vi "AS3_Spektrometer.vi"() -> ()   [LabVIEW 2013]
uses:
  subVIs_AS3_Spektrometer/ADC.vi
  subVIs_AS3_Spektrometer/readoutport.vi
panel:
  in  "Integration Time [s] 2":dbl=0.1
  in  "x-axis spectrum":cluster{dbl, dbl}(slide)={0.0, 3.6363636363636362} scale=0.0..10.0
  out "Camera NOT yet ready":bool
  in  "Leave Program":bool
  in  "Tab Control":T1(tab)=enum."Spectrum"
  in  "Autoscale Temperature":bool
  out "Temperature":cluster{dbl[], dbl[]}(graph)={[0.0, 0.25, 0.5, 0.75, 1.0, 1.25, 1.5, 1.75], [-30.0, -30.0, -30.0, -30.0, -30.0, -30.0, -30.0, -30.0]}
  in  "Temperature [°C]":dbl=-30.0
  out "Current Temperature [°C]":dbl=-30.0
  in  "Read Temperature":bool
  in  "stop 1":bool
  in  "Maximum Temperature Scale":dbl=-20.0
  in  "Minimum Temperature Scale":dbl=-40.0
  in  "Plot last 10 Seconds only":bool
  out "pixel scale":dbl[](array[numeric])=[0.0, 1.0, 2.0, 3.0, 4.0, 5.0, 6.0, 7.0, 8.0, 9.0, 10.0, 11.0, 12.0, 13.0, 14.0, 15.0, 16.0, 17.0, 18.0, 19.0, 20.0, 21.0, 22.0, 23.0, 24.0, 25.0, 26.0, 27.0, 28.0, 29.0, 30.0, 31.0, 32.0, 33.0, 34.0, 35.0, 36.0, 37.0, 38.0, 39.0, 40.0, 41.0, 42.0, 43.0, 44.0, 45.0, 46.0, 47.0, 48.0, 49.0, 50.0, 51.0, 52.0, 53.0, 54.0, 55.0, 56.0, 57.0, 58.0, 59.0, 60.0, 61.0, 62.0, 63.0, 64.0, 65.0, 66.0, 67.0, 68.0, 69.0, 70.0, 71.0, 72.0, 73.0, 74.0, 75.0, 76.0, 77.0, 78.0, 79.0, 80.0, 81.0, 82.0, 83.0, 84.0, 85.0, 86.0, 87.0, 88.0, 89.0, 90.0, 91.0, 92.0, 93.0, 94.0, 95.0, 96.0, 97.0, 98.0, 99.0, 100.0, 101.0, 102.0, 103.0, 104.0, 105.0, 106.0, 107.0, 108.0, 109.0, 110.0, 111.0, 112.0, 113.0, 114.0, 115.0, 116.0, 117.0, 118.0, 119.0, 120.0, 121.0, 122.0, 123.0, 124.0, 125.0, 126.0, 127.0, 128.0, 129.0, 130.0, 131.0, 132.0, 133.0, 134.0, 135.0, 136.0, 137.0, 138.0, 139.0, 140.0, 141.0, 142.0, 143.0, 144.0, 145.0, 146.0, 147.0, 148.0, 149.0, 150.0, 151.0, 152.0, 153.0, 154.0, 155.0, 156.0, 157.0, 158.0, 159.0, 160.0, 161.0, 162.0, 163.0, 164.0, 165.0, 166.0, 167.0, 168.0, 169.0, 170.0, 171.0, 172.0, 173.0, 174.0, 175.0, 176.0, 177.0, 178.0, 179.0, 180.0, 181.0, 182.0, 183.0, 184.0, 185.0, 186.0, 187.0, 188.0, 189.0, 190.0, 191.0, 192.0, 193.0, 194.0, 195.0, 196.0, 197.0, 198.0, 199.0, 200.0, 201.0, 202.0, 203.0, 204.0, 205.0, 206.0, 207.0, 208.0, 209.0, 210.0, 211.0, 212.0, 213.0, 214.0, 215.0, 216.0, 217.0, 218.0, 219.0, 220.0, 221.0, 222.0, 223.0, 224.0, 225.0, 226.0, 227.0, 228.0, 229.0, 230.0, 231.0, 232.0, 233.0, 234.0, 235.0, 236.0, 237.0, 238.0, 239.0, 240.0, 241.0, 242.0, 243.0, 244.0, 245.0, 246.0, 247.0, 248.0, 249.0, 250.0, 251.0, 252.0, 253.0, 254.0, 255.0, 256.0, 257.0, 258.0, 259.0, 260.0, 261.0, 262.0, 263.0, 264.0, 265.0, 266.0, 267.0, 268.0, 269.0, 270.0, 271.0, 272.0, 273.0, 274.0, 275.0, 276.0, 277.0, 278.0, 279.0, 280.0, 281.0, 282.0, 283.0, 284.0, 285.0, 286.0, 287.0, 288.0, 289.0, 290.0, 291.0, 292.0, 293.0, 294.0, 295.0, 296.0, 297.0, 298.0, 299.0, 300.0, 301.0, 302.0, 303.0, 304.0, 305.0, 306.0, 307.0, 308.0, 309.0, 310.0, 311.0, 312.0, 313.0, 314.0, 315.0, 316.0, 317.0, 318.0, 319.0, 320.0, 321.0, 322.0, 323.0, 324.0, 325.0, 326.0, 327.0, 328.0, 329.0, 330.0, 331.0, 332.0, 333.0, 334.0, 335.0, 336.0, 337.0, 338.0, 339.0, 340.0, 341.0, 342.0, 343.0, 344.0, 345.0, 346.0, 347.0, 348.0, 349.0, 350.0, 351.0, 352.0, 353.0, 354.0, 355.0, 356.0, 357.0, 358.0, 359.0, 360.0, 361.0, 362.0, 363.0, 364.0, 365.0, 366.0, 367.0, 368.0, 369.0, 370.0, 371.0, 372.0, 373.0, 374.0, 375.0, 376.0, 377.0, 378.0, 379.0, 380.0, 381.0, 382.0, 383.0, 384.0, 385.0, 386.0, 387.0, 388.0, 389.0, 390.0, 391.0, 392.0, 393.0, 394.0, 395.0, 396.0, 397.0, 398.0, 399.0, 400.0, 401.0, 402.0, 403.0, 404.0, 405.0, 406.0, 407.0, 408.0, 409.0, 410.0, 411.0, 412.0, 413.0, 414.0, 415.0, 416.0, 417.0, 418.0, 419.0, 420.0, 421.0, 422.0, 423.0, 424.0, 425.0, 426.0, 427.0, 428.0, 429.0, 430.0, 431.0, 432.0, 433.0, 434.0, 435.0, 436.0, 437.0, 438.0, 439.0, 440.0, 441.0, 442.0, 443.0, 444.0, 445.0, 446.0, 447.0, 448.0, 449.0, 450.0, 451.0, 452.0, 453.0, 454.0, 455.0, 456.0, 457.0, 458.0, 459.0, 460.0, 461.0, 462.0, 463.0, 464.0, 465.0, 466.0, 467.0, 468.0, 469.0, 470.0, 471.0, 472.0, 473.0, 474.0, 475.0, 476.0, 477.0, 478.0, 479.0, 480.0, 481.0, 482.0, 483.0, 484.0, 485.0, 486.0, 487.0, 488.0, 489.0, 490.0, 491.0, 492.0, 493.0, 494.0, 495.0, 496.0, 497.0, 498.0, 499.0, 500.0, 501.0, 502.0, 503.0, 504.0, 505.0, 506.0, 507.0, 508.0, 509.0, 510.0, 511.0, 512.0, 513.0, 514.0, 515.0, 516.0, 517.0, 518.0, 519.0, 520.0, 521.0, 522.0, 523.0, 524.0, 525.0, 526.0, 527.0, 528.0, 529.0, 530.0, 531.0, 532.0, 533.0, 534.0, 535.0, 536.0, 537.0, 538.0, 539.0, 540.0, 541.0, 542.0, 543.0, 544.0, 545.0, 546.0, 547.0, 548.0, 549.0, 550.0, 551.0, 552.0, 553.0, 554.0, 555.0, 556.0, 557.0, 558.0, 559.0, 560.0, 561.0, 562.0, 563.0, 564.0, 565.0, 566.0, 567.0, 568.0, 569.0, 570.0, 571.0, 572.0, 573.0, 574.0, 575.0, 576.0, 577.0, 578.0, 579.0, 580.0, 581.0, 582.0, 583.0, 584.0, 585.0, 586.0, 587.0, 588.0, 589.0, 590.0, 591.0, 592.0, 593.0, 594.0, 595.0, 596.0, 597.0, 598.0, 599.0, 600.0, 601.0, 602.0, 603.0, 604.0, 605.0, 606.0, 607.0, 608.0, 609.0, 610.0, 611.0, 612.0, 613.0, 614.0, 615.0, 616.0, 617.0, 618.0, 619.0, 620.0, 621.0, 622.0, 623.0, 624.0, 625.0, 626.0, 627.0, 628.0, 629.0, 630.0, 631.0, 632.0, 633.0, 634.0, 635.0, 636.0, 637.0, 638.0, 639.0, 640.0, 641.0, 642.0, 643.0, 644.0, 645.0, 646.0, 647.0, 648.0, 649.0, 650.0, 651.0, 652.0, 653.0, 654.0, 655.0, 656.0, 657.0, 658.0, 659.0, 660.0, 661.0, 662.0, 663.0, 664.0, 665.0, 666.0, 667.0, 668.0, 669.0, 670.0, 671.0, 672.0, 673.0, 674.0, 675.0, 676.0, 677.0, 678.0, 679.0, 680.0, 681.0, 682.0, 683.0, 684.0, 685.0, 686.0, 687.0, 688.0, 689.0, 690.0, 691.0, 692.0, 693.0, 694.0, 695.0, 696.0, 697.0, 698.0, 699.0, 700.0, 701.0, 702.0, 703.0, 704.0, 705.0, 706.0, 707.0, 708.0, 709.0, 710.0, 711.0, 712.0, 713.0, 714.0, 715.0, 716.0, 717.0, 718.0, 719.0, 720.0, 721.0, 722.0, 723.0, 724.0, 725.0, 726.0, 727.0, 728.0, 729.0, 730.0, 731.0, 732.0, 733.0, 734.0, 735.0, 736.0, 737.0, 738.0, 739.0, 740.0, 741.0, 742.0, 743.0, 744.0, 745.0, 746.0, 747.0, 748.0, 749.0, 750.0, 751.0, 752.0, 753.0, 754.0, 755.0, 756.0, 757.0, 758.0, 759.0, 760.0, 761.0, 762.0, 763.0, 764.0, 765.0, 766.0, 767.0, 768.0, 769.0, 770.0, 771.0, 772.0, 773.0, 774.0, 775.0, 776.0, 777.0, 778.0, 779.0, 780.0, 781.0, 782.0, 783.0, 784.0, 785.0, 786.0, 787.0, 788.0, 789.0, 790.0, 791.0, 792.0, 793.0, 794.0, 795.0, 796.0, 797.0, 798.0, 799.0, 800.0, 801.0, 802.0, 803.0, 804.0, 805.0, 806.0, 807.0, 808.0, 809.0, 810.0, 811.0, 812.0, 813.0, 814.0, 815.0, 816.0, 817.0, 818.0, 819.0, 820.0, 821.0, 822.0, 823.0, 824.0, 825.0, 826.0, 827.0, 828.0, 829.0, 830.0, 831.0, 832.0, 833.0, 834.0, 835.0, 836.0, 837.0, 838.0, 839.0, 840.0, 841.0, 842.0, 843.0, 844.0, 845.0, 846.0, 847.0, 848.0, 849.0, 850.0, 851.0, 852.0, 853.0, 854.0, 855.0, 856.0, 857.0, 858.0, 859.0, 860.0, 861.0, 862.0, 863.0, 864.0, 865.0, 866.0, 867.0, 868.0, 869.0, 870.0, 871.0, 872.0, 873.0, 874.0, 875.0, 876.0, 877.0, 878.0, 879.0, 880.0, 881.0, 882.0, 883.0, 884.0, 885.0, 886.0, 887.0, 888.0, 889.0, 890.0, 891.0, 892.0, 893.0, 894.0, 895.0, 896.0, 897.0, 898.0, 899.0, 900.0, 901.0, 902.0, 903.0, 904.0, 905.0, 906.0, 907.0, 908.0, 909.0, 910.0, 911.0, 912.0, 913.0, 914.0, 915.0, 916.0, 917.0, 918.0, 919.0, 920.0, 921.0, 922.0, 923.0, 924.0, 925.0, 926.0, 927.0, 928.0, 929.0, 930.0, 931.0, 932.0, 933.0, 934.0, 935.0, 936.0, 937.0, 938.0, 939.0, 940.0, 941.0, 942.0, 943.0, 944.0, 945.0, 946.0, 947.0, 948.0, 949.0, 950.0, 951.0, 952.0, 953.0, 954.0, 955.0, 956.0, 957.0, 958.0, 959.0, 960.0, 961.0, 962.0, 963.0, 964.0, 965.0, 966.0, 967.0, 968.0, 969.0, 970.0, 971.0, 972.0, 973.0, 974.0, 975.0, 976.0, 977.0, 978.0, 979.0, 980.0, 981.0, 982.0, 983.0, 984.0, 985.0, 986.0, 987.0, 988.0, 989.0, 990.0, 991.0, 992.0, 993.0, 994.0, 995.0, 996.0, 997.0, 998.0, 999.0, 1000.0, 1001.0, 1002.0, 1003.0, 1004.0, 1005.0, 1006.0, 1007.0, 1008.0, 1009.0, 1010.0, 1011.0, 1012.0, 1013.0, 1014.0, 1015.0, 1016.0, 1017.0, 1018.0, 1019.0, 1020.0, 1021.0, 1022.0, 1023.0, 1024.0, 1025.0, 1026.0, 1027.0, 1028.0, 1029.0, 1030.0, 1031.0, 1032.0, 1033.0, 1034.0, 1035.0, 1036.0, 1037.0, 1038.0, 1039.0, 1040.0, 1041.0, 1042.0, 1043.0, 1044.0, 1045.0, 1046.0, 1047.0, 1048.0, 1049.0, 1050.0, 1051.0, 1052.0, 1053.0, 1054.0, 1055.0, 1056.0, 1057.0, 1058.0, 1059.0, 1060.0, 1061.0, 1062.0, 1063.0, 1064.0, 1065.0, 1066.0, 1067.0, 1068.0, 1069.0, 1070.0, 1071.0, 1072.0, 1073.0, 1074.0, 1075.0, 1076.0, 1077.0, 1078.0, 1079.0, 1080.0, 1081.0, 1082.0, 1083.0, 1084.0, 1085.0, 1086.0, 1087.0, 1088.0, 1089.0, 1090.0, 1091.0, 1092.0, 1093.0, 1094.0, 1095.0, 1096.0, 1097.0, 1098.0, 1099.0, 1100.0, 1101.0, 1102.0, 1103.0, 1104.0, 1105.0, 1106.0, 1107.0, 1108.0, 1109.0, 1110.0, 1111.0, 1112.0, 1113.0, 1114.0, 1115.0, 1116.0, 1117.0, 1118.0, 1119.0, 1120.0, 1121.0, 1122.0, 1123.0, 1124.0, 1125.0, 1126.0, 1127.0, 1128.0, 1129.0, 1130.0, 1131.0, 1132.0, 1133.0, 1134.0, 1135.0, 1136.0, 1137.0, 1138.0, 1139.0, 1140.0, 1141.0, 1142.0, 1143.0, 1144.0, 1145.0, 1146.0, 1147.0, 1148.0, 1149.0, 1150.0, 1151.0, 1152.0, 1153.0, 1154.0, 1155.0, 1156.0, 1157.0, 1158.0, 1159.0, 1160.0, 1161.0, 1162.0, 1163.0, 1164.0, 1165.0, 1166.0, 1167.0, 1168.0, 1169.0, 1170.0, 1171.0, 1172.0, 1173.0, 1174.0, 1175.0, 1176.0, 1177.0, 1178.0, 1179.0, 1180.0, 1181.0, 1182.0, 1183.0, 1184.0, 1185.0, 1186.0, 1187.0, 1188.0, 1189.0, 1190.0, 1191.0, 1192.0, 1193.0, 1194.0, 1195.0, 1196.0, 1197.0, 1198.0, 1199.0, 1200.0, 1201.0, 1202.0, 1203.0, 1204.0, 1205.0, 1206.0, 1207.0, 1208.0, 1209.0, 1210.0, 1211.0, 1212.0, 1213.0, 1214.0, 1215.0, 1216.0, 1217.0, 1218.0, 1219.0, 1220.0, 1221.0, 1222.0, 1223.0, 1224.0, 1225.0, 1226.0, 1227.0, 1228.0, 1229.0, 1230.0, 1231.0, 1232.0, 1233.0, 1234.0, 1235.0, 1236.0, 1237.0, 1238.0, 1239.0, 1240.0, 1241.0, 1242.0, 1243.0, 1244.0, 1245.0, 1246.0, 1247.0, 1248.0, 1249.0, 1250.0, 1251.0, 1252.0, 1253.0, 1254.0, 1255.0, 1256.0, 1257.0, 1258.0, 1259.0, 1260.0, 1261.0, 1262.0, 1263.0, 1264.0, 1265.0, 1266.0, 1267.0, 1268.0, 1269.0, 1270.0, 1271.0, 1272.0, 1273.0, 1274.0, 1275.0, 1276.0, 1277.0, 1278.0, 1279.0, 1280.0, 1281.0, 1282.0, 1283.0, 1284.0, 1285.0, 1286.0, 1287.0, 1288.0, 1289.0, 1290.0, 1291.0, 1292.0, 1293.0, 1294.0, 1295.0, 1296.0, 1297.0, 1298.0, 1299.0, 1300.0, 1301.0, 1302.0, 1303.0, 1304.0, 1305.0, 1306.0, 1307.0, 1308.0, 1309.0, 1310.0, 1311.0, 1312.0, 1313.0, 1314.0, 1315.0, 1316.0, 1317.0, 1318.0, 1319.0, 1320.0, 1321.0, 1322.0, 1323.0, 1324.0, 1325.0, 1326.0, 1327.0, 1328.0, 1329.0, 1330.0, 1331.0, 1332.0, 1333.0, 1334.0, 1335.0, 1336.0, 1337.0, 1338.0, 1339.0]
  in  "Substract\nBackground":bool
  in  "Save Background":bool
  in  "Save Raw Data":bool
  in  "Change\nSettings":bool
  in  "Binning 1":u32(ring)=4 items=["1"=1, "2"=2, "4"=4, "10"=10]
  in  "Use Cursors":bool
  out "Current Loop":i32=1
  in  "Number of Averages":i32=1
  in  "Integration Time [s]":dbl=0.1
  in  "Scales of Full Chip Plot":T2={"X Max"=335.0, "Y Min"=1.0, "X Min"=1.0, "Y Max"=100.0}
  out "Full Chip Plot":dbl[][](graph)
  in  "stop 2":bool
  in  "Read Chip":bool
  out "ROI Parameters":T3={"X Start"=1, "X End"=1340, "Binning X"=4, "Y Start"=1, "Y End"=400, "Binning Y"=4}
  out "Plot Area":T4={"X min"=1.0, "Y min"=1.0, "X max"=335.0, "Y max"=100.0}
  out "Background Array":dbl[][](array[numeric])
  out "Binned Array 2":dbl[][](array[numeric])
  out "Binned Array 4":dbl[][](array[numeric])
  out "Binned Array 10":dbl[][](array[numeric])
  out "background\nspectrum":dbl[](array[numeric])=[4222.0, 3418.0, 3505.0, 3499.0, 3504.0, 3534.0, 3534.0, 3535.0, 3553.0, 3573.0, 3572.0, 3586.0, 3578.0, 3565.0, 3611.0, 3604.0, 3594.0, 3602.0, 3612.0, 3618.0, 3582.0, 3611.0, 3621.0, 3593.0, 3627.0, 3600.0, 3612.0, 3606.0, 3619.0, 3608.0, 3605.0, 3624.0, 3652.0, 3628.0, 3629.0, 3636.0, 3634.0, 3613.0, 3642.0, 3619.0, 3614.0, 3630.0, 3655.0, 3627.0, 3624.0, 3651.0, 3615.0, 3623.0, 3644.0, 3616.0, 3640.0, 3644.0, 3617.0, 3634.0, 3634.0, 3612.0, 3643.0, 3617.0, 3610.0, 3629.0, 3638.0, 3637.0, 3618.0, 3617.0, 3617.0, 3638.0, 3608.0, 3634.0, 3616.0, 3616.0, 3606.0, 3650.0, 3625.0, 3605.0, 3637.0, 3602.0, 3622.0, 3631.0, 3613.0, 3618.0, 3635.0, 3615.0, 3616.0, 3626.0, 3628.0, 3620.0, 3617.0, 3625.0, 3641.0, 3628.0, 3633.0, 3630.0, 3644.0, 3634.0, 3629.0, 3633.0, 3617.0, 3642.0, 3631.0, 3643.0, 3649.0, 3637.0, 3640.0, 3637.0, 3599.0, 3622.0, 3643.0, 3643.0, 3644.0, 3641.0, 3618.0, 3632.0, 3625.0, 3628.0, 3629.0, 3620.0, 3625.0, 3638.0, 3639.0, 3619.0, 3631.0, 3636.0, 3632.0, 3633.0, 3621.0, 3629.0, 3635.0, 3605.0, 3623.0, 3630.0, 3614.0, 3648.0, 3627.0, 3609.0, 3637.0, 3595.0, 3645.0, 3635.0, 3639.0, 3624.0, 3619.0, 3614.0, 3622.0, 3616.0, 3607.0, 3606.0, 3645.0, 3624.0, 3624.0, 3641.0, 3604.0, 3624.0, 3627.0, 3628.0, 3639.0, 3620.0, 3614.0, 3639.0, 3644.0, 3627.0, 3653.0, 3611.0, 3639.0, 3639.0, 3629.0, 3616.0, 3650.0, 3620.0, 3646.0, 3619.0, 3611.0, 3642.0, 3627.0, 3631.0, 3620.0, 3630.0, 3618.0, 3641.0, 3621.0, 3628.0, 3638.0, 3611.0, 3622.0, 3634.0, 3633.0, 3600.0, 3643.0, 3641.0, 3645.0, 3644.0, 3612.0, 3632.0, 3651.0, 3644.0, 3638.0, 3625.0, 3640.0, 3622.0, 3629.0, 3631.0, 3629.0, 3615.0, 3612.0, 3613.0, 3611.0, 3596.0, 3615.0, 3603.0, 3638.0, 3641.0, 3630.0, 3607.0, 3629.0, 3612.0, 3622.0, 3646.0, 3641.0, 3605.0, 3625.0, 3621.0, 3633.0, 3630.0, 3615.0, 3634.0, 3644.0, 3626.0, 3613.0, 3636.0, 3631.0, 3617.0, 3640.0, 3613.0, 3652.0, 3630.0, 3606.0, 3623.0, 3641.0, 3611.0, 3627.0, 3627.0, 3635.0, 3639.0, 3636.0, 3626.0, 3625.0, 3642.0, 3660.0, 3617.0, 3637.0, 3630.0, 3628.0, 3613.0, 3624.0, 3633.0, 3635.0, 3630.0, 3652.0, 3649.0, 3631.0, 3599.0, 3622.0, 3634.0, 3632.0, 3606.0, 3630.0, 3627.0, 3635.0, 3630.0, 3607.0, 3625.0, 3625.0, 3631.0, 3610.0, 3632.0, 3634.0, 3629.0, 3600.0, 3611.0, 3630.0, 3636.0, 3635.0, 3649.0, 3636.0, 3622.0, 3637.0, 3613.0, 3621.0, 3616.0, 3659.0, 3641.0, 3625.0, 3608.0, 3612.0, 3618.0, 3640.0, 3640.0, 3652.0, 3612.0, 3613.0, 3636.0, 3607.0, 3620.0, 3634.0, 3620.0, 3644.0, 3607.0, 3623.0, 3615.0, 3638.0, 3653.0, 3630.0, 3623.0, 3617.0, 3628.0, 3633.0, 3637.0, 3615.0, 3627.0, 3626.0, 3622.0, 3642.0, 3633.0, 3634.0, 3594.0, 3630.0, 3630.0, 3620.0, 3641.0, 3616.0, 3643.0, 3635.0, 3629.0, 3634.0, 3633.0, 3622.0, 3635.0, 3647.0, 3634.0, 3589.0, 3622.0, 3612.0, 3609.0, 3616.0, 3613.0, 3623.0, 3610.0, 3636.0, 3623.0, 3642.0, 3632.0, 3640.0, 3640.0, 3650.0, 3642.0, 3631.0, 3595.0, 3652.0, 3633.0, 3648.0, 3623.0, 3620.0, 3621.0, 3610.0, 3629.0, 3603.0, 3644.0, 3636.0, 3648.0, 3611.0, 3641.0, 3625.0, 3630.0, 3624.0, 3627.0, 3646.0, 3626.0, 3625.0, 3623.0, 3641.0, 3628.0, 3622.0, 3608.0, 3640.0, 3593.0, 3614.0, 3634.0, 3625.0, 3617.0, 3618.0, 3599.0, 3653.0, 3632.0, 3608.0, 3622.0, 3620.0, 3638.0, 3625.0, 3636.0, 3654.0, 3621.0, 3624.0, 3617.0, 3611.0, 3614.0, 3623.0, 3624.0, 3621.0, 3588.0, 3624.0, 3633.0, 3623.0, 3620.0, 3641.0, 3631.0, 3630.0, 3621.0, 3624.0, 3630.0, 3631.0, 3620.0, 3635.0, 3650.0, 3629.0, 3631.0, 3631.0, 3614.0, 3636.0, 3633.0, 3629.0, 3641.0, 3623.0, 3648.0, 3652.0, 3626.0, 3648.0, 3623.0, 3624.0, 3658.0, 3651.0, 3609.0, 3613.0, 3640.0, 3612.0, 3614.0, 3632.0, 3642.0, 3627.0, 3643.0, 3622.0, 3625.0, 3637.0, 3649.0, 3639.0, 3629.0, 3628.0, 3633.0, 3633.0, 3624.0, 3626.0, 3625.0, 3615.0, 3629.0, 3627.0, 3636.0, 3615.0, 3631.0, 3611.0, 3646.0, 3642.0, 3631.0, 3622.0, 3597.0, 3609.0, 3616.0, 3617.0, 3633.0, 3626.0, 3630.0, 3615.0, 3609.0, 3620.0, 3637.0, 3619.0, 3643.0, 3645.0, 3638.0, 3629.0, 3634.0, 3627.0, 3633.0, 3628.0, 3626.0, 3636.0, 3646.0, 3626.0, 3634.0, 3627.0, 3639.0, 3605.0, 3634.0, 3622.0, 3619.0, 3633.0, 3597.0, 3625.0, 3626.0, 3628.0, 3602.0, 3633.0, 3615.0, 3634.0, 3598.0, 3636.0, 3628.0, 3619.0, 3622.0, 3633.0, 3638.0, 3622.0, 3622.0, 3641.0, 3614.0, 3632.0, 3631.0, 3635.0, 3624.0, 3633.0, 3617.0, 3635.0, 3625.0, 3637.0, 3631.0, 3620.0, 3646.0, 3634.0, 3636.0, 3638.0, 3620.0, 3627.0, 3615.0, 3627.0, 3628.0, 3624.0, 3611.0, 3615.0, 3638.0, 3624.0, 3634.0, 3631.0, 3633.0, 3609.0, 3654.0, 3626.0, 3635.0, 3632.0, 3623.0, 3618.0, 3619.0, 3604.0, 3634.0, 3613.0, 3637.0, 3642.0, 3612.0, 3626.0, 3625.0, 3616.0, 3636.0, 3626.0, 3643.0, 3642.0, 3633.0, 3637.0, 3609.0, 3615.0, 3621.0, 3626.0, 3641.0, 3623.0, 3627.0, 3637.0, 3608.0, 3604.0, 3626.0, 3612.0, 3621.0, 3624.0, 3623.0, 3616.0, 3634.0, 3658.0, 3612.0, 3635.0, 3615.0, 3659.0, 3624.0, 3630.0, 3637.0, 3607.0, 3630.0, 3630.0, 3621.0, 3616.0, 3635.0, 3648.0, 3617.0, 3633.0, 3605.0, 3625.0, 3645.0, 3601.0, 3620.0, 3626.0, 3632.0, 3639.0, 3642.0, 3620.0, 3624.0, 3644.0, 3646.0, 3614.0, 3623.0, 3607.0, 3630.0, 3627.0, 3615.0, 3637.0, 3593.0, 3609.0, 3641.0, 3629.0, 3627.0, 3644.0, 3637.0, 3637.0, 3642.0, 3626.0, 3626.0, 3639.0, 3632.0, 3635.0, 3623.0, 3611.0, 3629.0, 3629.0, 3626.0, 3630.0, 3624.0, 3622.0, 3623.0, 3626.0, 3622.0, 3625.0, 3620.0, 3635.0, 3624.0, 3629.0, 3636.0, 3650.0, 3601.0, 3616.0, 3629.0, 3615.0, 3624.0, 3615.0, 3608.0, 3655.0, 3612.0, 3622.0, 3598.0, 3618.0, 3629.0, 3658.0, 3605.0, 3613.0, 3655.0, 3596.0, 3629.0, 3633.0, 3615.0, 3631.0, 3639.0, 3626.0, 3615.0, 3622.0, 3630.0, 3630.0, 3620.0, 3640.0, 3621.0, 3628.0, 3625.0, 3619.0, 3614.0, 3634.0, 3624.0, 3610.0, 3627.0, 3629.0, 3620.0, 3659.0, 3631.0, 3645.0, 3624.0, 3637.0, 3635.0, 3627.0, 3632.0, 3623.0, 3612.0, 3631.0, 3622.0, 3643.0, 3619.0, 3638.0, 3635.0, 3616.0, 3637.0, 3619.0, 3635.0, 3632.0, 3619.0, 3638.0, 3628.0, 3641.0, 3623.0, 3637.0, 3644.0, 3633.0, 3630.0, 3642.0, 3620.0, 3643.0, 3623.0, 3637.0, 3627.0, 3638.0, 3621.0, 3622.0, 3641.0, 3618.0, 3625.0, 3630.0, 3615.0, 3626.0, 3648.0, 3646.0, 3636.0, 3620.0, 3637.0, 3643.0, 3620.0, 3653.0, 3627.0, 3590.0, 3626.0, 3614.0, 3626.0, 3608.0, 3627.0, 3624.0, 3638.0, 3632.0, 3627.0, 3670.0, 3625.0, 3620.0, 3627.0, 3635.0, 3638.0, 3617.0, 3644.0, 3629.0, 3638.0, 3629.0, 3635.0, 3618.0, 3624.0, 3627.0, 3637.0, 3614.0, 3623.0, 3626.0, 3635.0, 3612.0, 3640.0, 3639.0, 3619.0, 3597.0, 3647.0, 3628.0, 3621.0, 3642.0, 3649.0, 3609.0, 3609.0, 3640.0, 3630.0, 3635.0, 3628.0, 3603.0, 3628.0, 3599.0, 3621.0, 3646.0, 3661.0, 3613.0, 3641.0, 3640.0, 3637.0, 3635.0, 3621.0, 3653.0, 3623.0, 3626.0, 3630.0, 3609.0, 3618.0, 3627.0, 3618.0, 3614.0, 3626.0, 3629.0, 3624.0, 3633.0, 3628.0, 3618.0, 3619.0, 3631.0, 3608.0, 3620.0, 3646.0, 3632.0, 3625.0, 3644.0, 3630.0, 3638.0, 3608.0, 3633.0, 3635.0, 3619.0, 3636.0, 3636.0, 3620.0, 3621.0, 3621.0, 3613.0, 3613.0, 3635.0, 3643.0, 3628.0, 3629.0, 3643.0, 3632.0, 3645.0, 3613.0, 3652.0, 3640.0, 3627.0, 3627.0, 3622.0, 3624.0, 3629.0, 3630.0, 3614.0, 3645.0, 3609.0, 3615.0, 3629.0, 3623.0, 3637.0, 3623.0, 3634.0, 3624.0, 3631.0, 3615.0, 3621.0, 3645.0, 3622.0, 3613.0, 3621.0, 3615.0, 3627.0, 3638.0, 3646.0, 3632.0, 3654.0, 3614.0, 3626.0, 3630.0, 3627.0, 3624.0, 3627.0, 3621.0, 3648.0, 3630.0, 3620.0, 3635.0, 3623.0, 3608.0, 3618.0, 3620.0, 3656.0, 3629.0, 3604.0, 3645.0, 3627.0, 3612.0, 3641.0, 3644.0, 3637.0, 3633.0, 3628.0, 3624.0, 3638.0, 3624.0, 3628.0, 3628.0, 3618.0, 3621.0, 3646.0, 3620.0, 3643.0, 3660.0, 3634.0, 3624.0, 3611.0, 3621.0, 3632.0, 3622.0, 3604.0, 3649.0, 3625.0, 3624.0, 3635.0, 3650.0, 3616.0, 3629.0, 3633.0, 3627.0, 3622.0, 3615.0, 3632.0, 3638.0, 3624.0, 3638.0, 3634.0, 3627.0, 3620.0, 3631.0, 3621.0, 3619.0, 3637.0, 3629.0, 3636.0, 3620.0, 3623.0, 3614.0, 3657.0, 3629.0, 3633.0, 3604.0, 3616.0, 3631.0, 3624.0, 3601.0, 3640.0, 3642.0, 3643.0, 3629.0, 3649.0, 3641.0, 3647.0, 3628.0, 3612.0, 3651.0, 3628.0, 3631.0, 3635.0, 3640.0, 3650.0, 3616.0, 3647.0, 3635.0, 3652.0, 3629.0, 3612.0, 3620.0, 3628.0, 3630.0, 3639.0, 3629.0, 3625.0, 3632.0, 3617.0, 3639.0, 3629.0, 3622.0, 3658.0, 3616.0, 3652.0, 3638.0, 3612.0, 3624.0, 3607.0, 3646.0, 3619.0, 3640.0, 3611.0, 3641.0, 3629.0, 3602.0, 3630.0, 3608.0, 3630.0, 3631.0, 3611.0, 3629.0, 3604.0, 3637.0, 3638.0, 3633.0, 3642.0, 3622.0, 3631.0, 3608.0, 3620.0, 3626.0, 3630.0, 3627.0, 3619.0, 3618.0, 3607.0, 3626.0, 3634.0, 3627.0, 3636.0, 3621.0, 3637.0, 3629.0, 3608.0, 3642.0, 3640.0, 3607.0, 3615.0, 3594.0, 3633.0, 3615.0, 3612.0, 3629.0, 3650.0, 3619.0, 3650.0, 3625.0, 3610.0, 3635.0, 3632.0, 3633.0, 3629.0, 3631.0, 3640.0, 3622.0, 3638.0, 3614.0, 3638.0, 3629.0, 3622.0, 3646.0, 3614.0, 3614.0, 3617.0, 3640.0, 3623.0, 3610.0, 3612.0, 3623.0, 3632.0, 3622.0, 3651.0, 3624.0, 3623.0, 3641.0, 3645.0, 3634.0, 3651.0, 3622.0, 3627.0, 3625.0, 3620.0, 3617.0, 3617.0, 3646.0, 3629.0, 3621.0, 3630.0, 3613.0, 3621.0, 3645.0, 3634.0, 3631.0, 3635.0, 3651.0, 3620.0, 3620.0, 3633.0, 3628.0, 3632.0, 3623.0, 3636.0, 3615.0, 3595.0, 3626.0, 3638.0, 3623.0, 3620.0, 3642.0, 3621.0, 3621.0, 3625.0, 3611.0, 3633.0, 3616.0, 3623.0, 3632.0, 3645.0, 3613.0, 3611.0, 3623.0, 3633.0, 3619.0, 3624.0, 3639.0, 3599.0, 3640.0, 3627.0, 3606.0, 3628.0, 3644.0, 3622.0, 3607.0, 3637.0, 3618.0, 3630.0, 3613.0, 3614.0, 3631.0, 3612.0, 3637.0, 3613.0, 3641.0, 3636.0, 3633.0, 3621.0, 3628.0, 3633.0, 3623.0, 3654.0, 3632.0, 3601.0, 3623.0, 3621.0, 3643.0, 3648.0, 3642.0, 3610.0, 3608.0, 3633.0, 3604.0, 3611.0, 3634.0, 3620.0, 3633.0, 3627.0, 3611.0, 3630.0, 3601.0, 3622.0, 3631.0, 3608.0, 3620.0, 3620.0, 3615.0, 3642.0, 3613.0, 3627.0, 3621.0, 3617.0, 3617.0, 3633.0, 3620.0, 3612.0, 3625.0, 3660.0, 3649.0, 3629.0, 3630.0, 3616.0, 3630.0, 3631.0, 3642.0, 3615.0, 3622.0, 3625.0, 3622.0, 3629.0, 3628.0, 3609.0, 3623.0, 3617.0, 3615.0, 3639.0, 3619.0, 3631.0, 3611.0, 3609.0, 3618.0, 3641.0, 3617.0, 3605.0, 3634.0, 3623.0, 3606.0, 3638.0, 3624.0, 3629.0, 3648.0, 3600.0, 3630.0, 3613.0, 3627.0, 3615.0, 3621.0, 3626.0, 3617.0, 3650.0, 3625.0, 3597.0, 3620.0, 3611.0, 3621.0, 3619.0, 3633.0, 3620.0, 3630.0, 3634.0, 3644.0, 3626.0, 3641.0, 3639.0, 3629.0, 3618.0, 3623.0, 3628.0, 3624.0, 3603.0, 3627.0, 3631.0, 3647.0, 3639.0, 3636.0, 3632.0, 3631.0, 3629.0, 3635.0, 3625.0, 3643.0, 3619.0, 3618.0, 3632.0, 3631.0, 3606.0, 3626.0, 3633.0, 3638.0, 3622.0, 3629.0, 3607.0, 3630.0, 3614.0, 3627.0, 3646.0, 3625.0, 3624.0, 3623.0, 3632.0, 3606.0, 3614.0, 3629.0, 3619.0, 3629.0, 3631.0, 3621.0, 3633.0, 3608.0, 3644.0, 3620.0, 3621.0, 3620.0, 3633.0, 3610.0, 3625.0, 3634.0, 3638.0, 3615.0, 3626.0, 3631.0, 3629.0, 3632.0, 3614.0, 3604.0, 3608.0, 3609.0, 3606.0, 3648.0, 3654.0, 3619.0, 3665.0, 3614.0, 3607.0, 3632.0, 3639.0, 3604.0, 3624.0, 3637.0, 3634.0, 3624.0, 3636.0, 3628.0, 3639.0, 3618.0, 3631.0, 3610.0, 3629.0, 3638.0, 3612.0, 3624.0, 3628.0, 3648.0, 3629.0]
  out "Index 2":u32=1
  out "Index 1":u32=1
  out "Image Handle":u32=1
  out "back":dbl[][](array[numeric])
  in  "Comment":string="MCP \nNe mbar"
  in  "Save to Logbook":bool
  in  "Autoscale":bool=TRUE
  in  "Use latest\nEnergy Scale":bool
  in  "New Calibration":bool
  out "already calibrated?":bool=TRUE
  in  "stop 3":bool
  in  "Start Calibration":bool
  in  "calibration spectra":u16(ring)=2 items=["current spectrum"=1, "averaged spectrum"=2, "background spectrum"=4]
  in  "Number of\nAverages":i32=3
  out "Current\nLoop":i32=2
  out "normalized spectra":cluster{dbl[], dbl[]}[](graph)
  in  "Calibrate":bool
  in  "First Edge [eV]":dbl=100.0
  in  "Second Edge [eV]":dbl=72.8
  in  "Save second spectrum for calibration":bool
  in  "Save first spectrum for calibration":bool
  out "current spectrum":cluster{"Value":dbl[], "Value":dbl[]}[](graph)
  out "background spectrum":cluster{"Value":dbl[], dbl[]}[](graph)
  out "averaged spectrum":T5(graph)
  in  "Substract\nBackground 2":bool
  out "Energy Scale in eV":dbl[](array[numeric])=[56.2886283295992, 56.36666666666666, 56.44470500373413, 56.52274334080158, 56.60078167786905, 56.67882001493652, 56.756858352003974, 56.83489668907144, 56.9129350261389, 56.990973363206365, 57.06901170027383, 57.147050037341295, 57.225088374408756, 57.303126711476224, 57.381165048543686, 57.45920338561115, 57.53724172267861, 57.61528005974607, 57.69331839681354, 57.771356733881, 57.84939507094846, 57.92743340801593, 58.00547174508339, 58.08351008215085, 58.16154841921832, 58.23958675628578, 58.31762509335324, 58.395663430420704, 58.473701767488166, 58.551740104555634, 58.629778441623095, 58.70781677869056, 58.785855115758025, 58.86389345282549, 58.94193178989295, 59.019970126960416, 59.09800846402788, 59.17604680109534, 59.25408513816281, 59.33212347523027, 59.41016181229773, 59.48820014936519, 59.56623848643265, 59.64427682350012, 59.72231516056758, 59.800353497635044, 59.87839183470251, 59.95643017176997, 60.034468508837435, 60.1125068459049, 60.190545182972365, 60.268583520039826, 60.34662185710729, 60.42466019417475, 60.50269853124222, 60.58073686830968, 60.65877520537714, 60.73681354244461, 60.81485187951207, 60.89289021657953, 60.970928553647, 61.04896689071446, 61.12700522778192, 61.20504356484938, 61.283081901916844, 61.36112023898431, 61.439158576051774, 61.517196913119236, 61.595235250186704, 61.673273587254165, 61.75131192432163, 61.829350261389095, 61.907388598456556, 61.98542693552402, 62.063465272591486, 62.14150360965895, 62.21954194672641, 62.29758028379387, 62.37561862086133, 62.4536569579288, 62.53169529499626, 62.60973363206372, 62.68777196913119, 62.76581030619865, 62.843848643266114, 62.92188698033358, 62.99992531740104, 63.077963654468505, 63.156001991535966, 63.23404032860343, 63.312078665670896, 63.39011700273836, 63.46815533980582, 63.54619367687329, 63.62423201394075, 63.70227035100821, 63.78030868807568, 63.85834702514314, 63.9363853622106, 64.01442369927807, 64.09246203634552, 64.17050037341299, 64.24853871048046, 64.32657704754791, 64.40461538461538, 64.48265372168285, 64.5606920587503, 64.63873039581776, 64.71676873288524, 64.7948070699527, 64.87284540702015, 64.95088374408762, 65.02892208115509, 65.10696041822254, 65.18499875529001, 65.26303709235748, 65.34107542942493, 65.4191137664924, 65.49715210355987, 65.57519044062732, 65.65322877769479, 65.73126711476226, 65.80930545182972, 65.88734378889718, 65.96538212596465, 66.0434204630321, 66.12145880009957, 66.19949713716704, 66.2775354742345, 66.35557381130195, 66.43361214836943, 66.51165048543689, 66.58968882250434, 66.66772715957183, 66.74576549663928, 66.82380383370673, 66.9018421707742, 66.97988050784167, 67.05791884490912, 67.1359571819766, 67.21399551904406, 67.29203385611152, 67.37007219317898, 67.44811053024645, 67.5261488673139, 67.60418720438138, 67.68222554144884, 67.7602638785163, 67.83830221558377, 67.91634055265123, 67.99437888971869, 68.07241722678616, 68.15045556385363, 68.22849390092108, 68.30653223798855, 68.384570575056, 68.46260891212347, 68.54064724919094, 68.6186855862584, 68.69672392332586, 68.77476226039332, 68.85280059746079, 68.93083893452825, 69.00887727159571, 69.08691560866318, 69.16495394573064, 69.2429922827981, 69.32103061986557, 69.39906895693304, 69.47710729400049, 69.55514563106796, 69.63318396813543, 69.71122230520288, 69.78926064227035, 69.86729897933782, 69.94533731640527, 70.02337565347274, 70.10141399054021, 70.17945232760766, 70.25749066467513, 70.33552900174259, 70.41356733881005, 70.49160567587751, 70.56964401294498, 70.64768235001245, 70.7257206870799, 70.80375902414737, 70.88179736121484, 70.95983569828229, 71.03787403534976, 71.11591237241723, 71.19395070948468, 71.27198904655215, 71.35002738361962, 71.42806572068707, 71.50610405775454, 71.58414239482201, 71.66218073188946, 71.74021906895693, 71.8182574060244, 71.89629574309186, 71.97433408015932, 72.05237241722678, 72.13041075429425, 72.20844909136171, 72.28648742842917, 72.36452576549664, 72.44256410256409, 72.52060243963156, 72.59864077669903, 72.67667911376648, 72.75471745083395, 72.83275578790142, 72.91079412496887, 72.98883246203634, 73.06687079910381, 73.14490913617126, 73.22294747323873, 73.3009858103062, 73.37902414737366, 73.45706248444112, 73.53510082150859, 73.61313915857605, 73.69117749564352, 73.76921583271098, 73.84725416977844, 73.9252925068459, 74.00333084391336, 74.08136918098083, 74.15940751804828, 74.23744585511575, 74.31548419218322, 74.39352252925067, 74.47156086631814, 74.54959920338561, 74.62763754045307, 74.70567587752053, 74.783714214588, 74.86175255165546, 74.93979088872292, 75.0178292257904, 75.09586756285785, 75.17390589992532, 75.25194423699278, 75.32998257406024, 75.40802091112771, 75.48605924819518, 75.56409758526263, 75.6421359223301, 75.72017425939757, 75.79821259646502, 75.87625093353249, 75.95428927059994, 76.03232760766741, 76.11036594473487, 76.18840428180233, 76.2664426188698, 76.34448095593726, 76.42251929300473, 76.5005576300722, 76.57859596713965, 76.65663430420712, 76.73467264127459, 76.81271097834204, 76.89074931540951, 76.96878765247698, 77.04682598954443, 77.1248643266119, 77.20290266367937, 77.28094100074682, 77.35897933781429, 77.43701767488176, 77.51505601194921, 77.59309434901668, 77.67113268608414, 77.7491710231516, 77.82720936021907, 77.90524769728653, 77.983286034354, 78.06132437142145, 78.13936270848892, 78.21740104555639, 78.29543938262384, 78.37347771969131, 78.45151605675878, 78.52955439382623, 78.6075927308937, 78.68563106796117, 78.76366940502862, 78.84170774209609, 78.91974607916356, 78.99778441623101, 79.07582275329848, 79.15386109036595, 79.2318994274334, 79.30993776450087, 79.38797610156834, 79.4660144386358, 79.54405277570326, 79.62209111277072, 79.70012944983819, 79.77816778690564, 79.85620612397311, 79.93424446104058, 80.01228279810803, 80.0903211351755, 80.16835947224297, 80.24639780931042, 80.32443614637789, 80.40247448344536, 80.48051282051281, 80.55855115758028, 80.63658949464775, 80.7146278317152, 80.79266616878267, 80.87070450585014, 80.9487428429176, 81.02678117998506, 81.10481951705253, 81.18285785411999, 81.26089619118746, 81.33893452825492, 81.41697286532238, 81.49501120238985, 81.5730495394573, 81.65108787652477, 81.72912621359222, 81.80716455065969, 81.88520288772716, 81.96324122479461, 82.04127956186208, 82.11931789892955, 82.197356235997, 82.27539457306447, 82.35343291013194, 82.4314712471994, 82.50950958426687, 82.58754792133433, 82.66558625840179, 82.74362459546926, 82.82166293253673, 82.89970126960418, 82.97773960667165, 83.05577794373912, 83.13381628080657, 83.21185461787404, 83.2898929549415, 83.36793129200896, 83.44596962907642, 83.52400796614388, 83.60204630321135, 83.6800846402788, 83.75812297734628, 83.83616131441374, 83.9141996514812, 83.99223798854867, 84.07027632561613, 84.14831466268359, 84.22635299975106, 84.30439133681853, 84.38242967388598, 84.46046801095345, 84.53850634802092, 84.61654468508837, 84.69458302215584, 84.77262135922331, 84.85065969629076, 84.92869803335823, 85.0067363704257, 85.08477470749315, 85.16281304456062, 85.24085138162808, 85.31888971869554, 85.39692805576301, 85.47496639283047, 85.55300472989794, 85.63104306696539, 85.70908140403286, 85.78711974110033, 85.86515807816778, 85.94319641523525, 86.02123475230272, 86.09927308937017, 86.17731142643764, 86.25534976350511, 86.33338810057256, 86.41142643764003, 86.4894647747075, 86.56750311177495, 86.64554144884242, 86.72357978590989, 86.80161812297735, 86.87965646004481, 86.95769479711228, 87.03573313417974, 87.1137714712472, 87.19180980831466, 87.26984814538213, 87.34788648244958, 87.42592481951705, 87.50396315658452, 87.58200149365197, 87.66003983071944, 87.73807816778691, 87.81611650485436, 87.89415484192183, 87.9721931789893, 88.05023151605675, 88.12826985312422, 88.20630819019169, 88.28434652725915, 88.36238486432661, 88.44042320139408, 88.51846153846154, 88.596499875529, 88.67453821259647, 88.75257654966393, 88.8306148867314, 88.90865322379886, 88.98669156086632, 89.06472989793379, 89.14276823500124, 89.22080657206871, 89.29884490913616, 89.37688324620363, 89.4549215832711, 89.53295992033856, 89.61099825740602, 89.68903659447349, 89.76707493154095, 89.84511326860842, 89.92315160567588, 90.00118994274334, 90.0792282798108, 90.15726661687827, 90.23530495394573, 90.3133432910132, 90.39138162808067, 90.46941996514812, 90.54745830221559, 90.62549663928306, 90.70353497635051, 90.78157331341798, 90.85961165048543, 90.9376499875529, 91.01568832462037, 91.09372666168782, 91.1717649987553, 91.24980333582275, 91.32784167289022, 91.40588000995768, 91.48391834702514, 91.5619566840926, 91.63999502116008, 91.71803335822753, 91.796071695295, 91.87411003236247, 91.95214836942992, 92.03018670649739, 92.10822504356486, 92.18626338063231, 92.26430171769978, 92.34234005476725, 92.4203783918347, 92.49841672890217, 92.57645506596964, 92.6544934030371, 92.73253174010456, 92.81057007717202, 92.88860841423949, 92.96664675130694, 93.04468508837441, 93.12272342544188, 93.20076176250933, 93.2788000995768, 93.35683843664427, 93.43487677371172, 93.51291511077919, 93.59095344784666, 93.66899178491411, 93.74703012198158, 93.82506845904905, 93.9031067961165, 93.98114513318397, 94.05918347025144, 94.1372218073189, 94.21526014438636, 94.29329848145383, 94.37133681852129, 94.44937515558875, 94.52741349265622, 94.60545182972368, 94.68349016679115, 94.7615285038586, 94.83956684092607, 94.91760517799352, 94.99564351506099, 95.07368185212846, 95.15172018919591, 95.22975852626338, 95.30779686333085, 95.3858352003983, 95.46387353746577, 95.54191187453324, 95.6199502116007, 95.69798854866816, 95.77602688573563, 95.85406522280309, 95.93210355987055, 96.01014189693802, 96.08818023400548, 96.16621857107295, 96.24425690814041, 96.32229524520787, 96.40033358227534, 96.47837191934279, 96.55641025641026, 96.63444859347773, 96.71248693054518, 96.79052526761265, 96.8685636046801, 96.94660194174757, 97.02464027881504, 97.1026786158825, 97.18071695294996, 97.25875529001743, 97.33679362708489, 97.41483196415236, 97.49287030121982, 97.57090863828728, 97.64894697535475, 97.72698531242222, 97.80502364948967, 97.88306198655714, 97.9611003236246, 98.03913866069206, 98.11717699775953, 98.195215334827, 98.27325367189445, 98.35129200896192, 98.42933034602937, 98.50736868309684, 98.5854070201643, 98.66344535723177, 98.74148369429923, 98.81952203136669, 98.89756036843416, 98.97559870550162, 99.05363704256908, 99.13167537963655, 99.20971371670402, 99.28775205377147, 99.36579039083894, 99.4438287279064, 99.52186706497386, 99.59990540204133, 99.6779437391088, 99.75598207617625, 99.83402041324372, 99.91205875031119, 99.99009708737864, 100.06813542444611, 100.14617376151358, 100.22421209858103, 100.3022504356485, 100.38028877271596, 100.45832710978343, 100.53636544685088, 100.61440378391835, 100.69244212098582, 100.77048045805327, 100.84851879512074, 100.92655713218821, 101.00459546925566, 101.08263380632313, 101.1606721433906, 101.23871048045805, 101.31674881752552, 101.39478715459299, 101.47282549166044, 101.55086382872791, 101.62890216579538, 101.70694050286284, 101.7849788399303, 101.86301717699777, 101.94105551406523, 102.0190938511327, 102.09713218820015, 102.17517052526762, 102.25320886233507, 102.33124719940254, 102.40928553647001, 102.48732387353746, 102.56536221060493, 102.6434005476724, 102.72143888473985, 102.79947722180732, 102.87751555887479, 102.95555389594224, 103.03359223300971, 103.11163057007718, 103.18966890714464, 103.2677072442121, 103.34574558127957, 103.42378391834703, 103.5018222554145, 103.57986059248196, 103.65789892954942, 103.73593726661689, 103.81397560368436, 103.89201394075181, 103.97005227781928, 104.04809061488673, 104.1261289519542, 104.20416728902165, 104.28220562608912, 104.36024396315659, 104.43828230022405, 104.51632063729151, 104.59435897435898, 104.67239731142644, 104.7504356484939, 104.82847398556137, 104.90651232262883, 104.9845506596963, 105.06258899676376, 105.14062733383122, 105.21866567089869, 105.29670400796616, 105.37474234503361, 105.45278068210108, 105.53081901916855, 105.608857356236, 105.68689569330346, 105.76493403037094, 105.84297236743839, 105.92101070450585, 105.99904904157333, 106.07708737864078, 106.15512571570824, 106.2331640527757, 106.31120238984317, 106.38924072691063, 106.4672790639781, 106.54531740104557, 106.62335573811302, 106.70139407518049, 106.77943241224796, 106.85747074931541, 106.93550908638288, 107.01354742345035, 107.0915857605178, 107.16962409758527, 107.24766243465274, 107.3257007717202, 107.40373910878766, 107.48177744585513, 107.55981578292258, 107.63785411999004, 107.71589245705752, 107.79393079412498, 107.87196913119243, 107.9500074682599, 108.02804580532737, 108.10608414239482, 108.18412247946229, 108.26216081652976, 108.34019915359721, 108.41823749066468, 108.49627582773215, 108.5743141647996, 108.65235250186707, 108.73039083893454, 108.808429176002, 108.88646751306946, 108.96450585013693, 109.04254418720438, 109.12058252427185, 109.19862086133932, 109.27665919840678, 109.35469753547423, 109.43273587254171, 109.51077420960917, 109.58881254667662, 109.6668508837441, 109.74488922081156, 109.82292755787901, 109.90096589494648, 109.97900423201395, 110.0570425690814, 110.13508090614887, 110.21311924321634, 110.2911575802838, 110.36919591735126, 110.44723425441873, 110.52527259148619, 110.60331092855365, 110.68134926562112, 110.75938760268858, 110.83742593975605, 110.91546427682351, 110.99350261389097, 111.07154095095844, 111.1495792880259, 111.22761762509336, 111.30565596216081, 111.3836942992283, 111.46173263629575, 111.5397709733632, 111.61780931043069, 111.69584764749814, 111.7738859845656, 111.85192432163306, 111.92996265870053, 112.00800099576799, 112.08603933283545, 112.16407766990292, 112.24211600697038, 112.32015434403785, 112.39819268110531, 112.47623101817277, 112.55426935524024, 112.6323076923077, 112.71034602937516, 112.78838436644263, 112.8664227035101, 112.94446104057755, 113.02249937764502, 113.10053771471249, 113.17857605177994, 113.2566143888474, 113.33465272591488, 113.41269106298233, 113.49072940004979, 113.56876773711726, 113.64680607418472, 113.72484441125218, 113.80288274831965, 113.88092108538711, 113.95895942245457, 114.03699775952204, 114.1150360965895, 114.19307443365696, 114.27111277072443, 114.3491511077919, 114.42718944485935, 114.50522778192682, 114.58326611899429, 114.66130445606174, 114.73934279312921, 114.81738113019668, 114.89541946726413, 114.97345780433159, 115.05149614139907, 115.12953447846652, 115.20757281553398, 115.28561115260146, 115.36364948966892, 115.44168782673637, 115.51972616380384, 115.5977645008713, 115.67580283793876, 115.75384117500623, 115.8318795120737, 115.90991784914115, 115.98795618620862, 116.06599452327609, 116.14403286034354, 116.22207119741101, 116.30010953447848, 116.37814787154593, 116.4561862086134, 116.53422454568087, 116.61226288274833, 116.6903012198158, 116.76833955688326, 116.84637789395072, 116.92441623101817, 117.00245456808565, 117.08049290515311, 117.15853124222056, 117.23656957928803, 117.3146079163555, 117.39264625342295, 117.47068459049042, 117.54872292755789, 117.62676126462534, 117.70479960169281, 117.78283793876028, 117.86087627582774, 117.9389146128952, 118.01695294996267, 118.09499128703013, 118.1730296240976, 118.25106796116506, 118.32910629823252, 118.40714463529999, 118.48518297236745, 118.56322130943491, 118.64125964650236, 118.71929798356985, 118.7973363206373, 118.87537465770475, 118.95341299477224, 119.03145133183969, 119.10948966890714, 119.18752800597461, 119.26556634304208, 119.34360468010954, 119.421643017177, 119.49968135424447, 119.57771969131193, 119.6557580283794, 119.73379636544686, 119.81183470251432, 119.88987303958179, 119.96791137664925, 120.04594971371671, 120.12398805078418, 120.20202638785165, 120.2800647249191, 120.35810306198657, 120.43614139905404, 120.51417973612149, 120.59221807318895, 120.67025641025643, 120.74829474732388, 120.82633308439134, 120.90437142145882, 120.98240975852627, 121.06044809559373, 121.1384864326612, 121.21652476972866, 121.29456310679612, 121.37260144386359, 121.45063978093106, 121.52867811799851, 121.60671645506598, 121.68475479213345, 121.7627931292009, 121.84083146626837, 121.91886980333584, 121.99690814040329, 122.07494647747076, 122.15298481453823, 122.23102315160568, 122.30906148867315, 122.38709982574062, 122.46513816280807, 122.54317649987553, 122.62121483694301, 122.69925317401047, 122.77729151107792, 122.85532984814539, 122.93336818521286, 123.01140652228031, 123.08944485934778, 123.16748319641525, 123.2455215334827, 123.32355987055017, 123.40159820761764, 123.47963654468509, 123.55767488175256, 123.63571321882003, 123.71375155588748, 123.79178989295495, 123.86982823002242, 123.94786656708987, 124.02590490415734, 124.10394324122481, 124.18198157829227, 124.26001991535972, 124.3380582524272, 124.41609658949466, 124.49413492656211, 124.5721732636296, 124.65021160069705, 124.7282499377645, 124.80628827483197, 124.88432661189944, 124.9623649489669, 125.04040328603436, 125.11844162310183, 125.19647996016928, 125.27451829723675, 125.35255663430422, 125.43059497137168, 125.50863330843914, 125.58667164550661, 125.66470998257407, 125.74274831964154, 125.820786656709, 125.89882499377646, 125.97686333084393, 126.0549016679114, 126.13294000497885, 126.2109783420463, 126.28901667911379, 126.36705501618124, 126.4450933532487, 126.52313169031616, 126.60117002738363, 126.67920836445109, 126.75724670151855, 126.83528503858602, 126.91332337565348, 126.99136171272094, 127.06940004978841, 127.14743838685587, 127.22547672392334, 127.3035150609908, 127.38155339805826, 127.45959173512573, 127.5376300721932, 127.61566840926065, 127.69370674632812, 127.77174508339559, 127.84978342046304, 127.9278217575305, 128.00586009459798, 128.08389843166543, 128.1619367687329, 128.23997510580037, 128.31801344286782, 128.39605177993528, 128.47409011700273, 128.5521284540702, 128.63016679113767, 128.70820512820512, 128.7862434652726, 128.86428180234006, 128.9423201394075, 129.020358476475, 129.09839681354245, 129.1764351506099, 129.2544734876774, 129.33251182474484, 129.4105501618123, 129.48858849887978, 129.56662683594723, 129.6446651730147, 129.72270351008217, 129.80074184714962, 129.87878018421708, 129.95681852128456, 130.03485685835201, 130.11289519541947, 130.19093353248695, 130.2689718695544, 130.34701020662186, 130.42504854368934, 130.5030868807568, 130.58112521782425, 130.65916355489173, 130.7372018919592, 130.81524022902664, 130.89327856609412, 130.97131690316158, 131.04935524022903, 131.12739357729652, 131.20543191436397, 131.28347025143142, 131.3615085884989, 131.43954692556636, 131.51758526263382, 131.5956235997013, 131.67366193676875, 131.7517002738362, 131.82973861090366, 131.90777694797114, 131.9858152850386, 132.06385362210605, 132.1418919591735, 132.219930296241, 132.29796863330844, 132.3760069703759, 132.45404530744338, 132.53208364451083, 132.6101219815783, 132.68816031864577, 132.76619865571323, 132.84423699278068, 132.92227532984816, 133.00031366691562, 133.07835200398307, 133.15639034105055, 133.234428678118, 133.31246701518546, 133.39050535225294, 133.4685436893204, 133.54658202638785, 133.62462036345534, 133.7026587005228, 133.78069703759024, 133.85873537465773, 133.93677371172518, 134.01481204879263, 134.09285038586012, 134.17088872292757, 134.24892705999503, 134.3269653970625, 134.40500373412996, 134.48304207119742, 134.5610804082649, 134.63911874533235, 134.7171570823998, 134.7951954194673, 134.87323375653474, 134.9512720936022, 135.02931043066968, 135.10734876773714, 135.1853871048046, 135.26342544187207, 135.34146377893953, 135.41950211600698, 135.49754045307444, 135.5755787901419, 135.65361712720937, 135.73165546427683, 135.80969380134428, 135.88773213841176, 135.96577047547922, 136.04380881254667, 136.12184714961415, 136.1998854866816, 136.27792382374906, 136.35596216081655, 136.434000497884, 136.51203883495145, 136.59007717201894, 136.6681155090864, 136.74615384615385, 136.82419218322133, 136.90223052028878, 136.98026885735624, 137.05830719442372, 137.13634553149117, 137.21438386855863, 137.2924222056261, 137.37046054269356, 137.44849887976102, 137.5265372168285, 137.60457555389596, 137.6826138909634, 137.7606522280309, 137.83869056509835, 137.9167289021658, 137.99476723923328, 138.07280557630074, 138.1508439133682, 138.22888225043567, 138.30692058750313, 138.38495892457058, 138.46299726163807, 138.54103559870552, 138.61907393577297, 138.69711227284046, 138.7751506099079, 138.85318894697537, 138.93122728404285, 139.00926562111027, 139.08730395817776, 139.16534229524524, 139.24338063231266, 139.32141896938015, 139.39945730644763, 139.47749564351506, 139.55553398058254, 139.63357231765002, 139.71161065471745, 139.78964899178493, 139.86768732885238, 139.94572566591984, 140.02376400298732, 140.10180234005477, 140.17984067712223, 140.2578790141897, 140.33591735125717, 140.41395568832462, 140.4919940253921, 140.57003236245956, 140.648070699527, 140.7261090365945, 140.80414737366195, 140.8821857107294, 140.96022404779688, 141.03826238486434, 141.1163007219318, 141.19433905899928, 141.27237739606673, 141.35041573313418, 141.42845407020167, 141.50649240726912, 141.58453074433658, 141.66256908140406, 141.7406074184715, 141.81864575553897, 141.89668409260645, 141.9747224296739, 142.05276076674136, 142.13079910380884, 142.2088374408763, 142.28687577794375, 142.36491411501123, 142.44295245207869, 142.52099078914614, 142.59902912621362, 142.67706746328105, 142.75510580034853, 142.833144137416, 142.91118247448344, 142.98922081155092, 143.0672591486184, 143.14529748568583, 143.2233358227533, 143.3013741598208, 143.37941249688822, 143.4574508339557, 143.53548917102316, 143.6135275080906, 143.6915658451581, 143.76960418222555, 143.847642519293, 143.9256808563605, 144.00371919342794, 144.0817575304954, 144.15979586756288, 144.23783420463033, 144.3158725416978, 144.39391087876527, 144.47194921583272, 144.54998755290018, 144.62802588996766, 144.7060642270351, 144.78410256410257, 144.86214090117005, 144.9401792382375, 145.01821757530496, 145.09625591237244, 145.1742942494399, 145.25233258650735, 145.33037092357483, 145.4084092606423, 145.48644759770974, 145.56448593477722, 145.64252427184468, 145.72056260891213, 145.79860094597962, 145.87663928304707, 145.95467762011452, 146.032715957182, 146.11075429424946, 146.18879263131691, 146.2668309683844, 146.34486930545182, 146.4229076425193, 146.5009459795868, 146.5789843166542, 146.6570226537217, 146.73506099078918, 146.8130993278566, 146.8911376649241, 146.96917600199157, 147.047214339059, 147.12525267612648, 147.20329101319393, 147.2813293502614, 147.35936768732887, 147.43740602439632, 147.51544436146378, 147.59348269853126, 147.67152103559872, 147.74955937266617, 147.82759770973365, 147.9056360468011, 147.98367438386856, 148.06171272093604, 148.1397510580035, 148.21778939507095, 148.29582773213843, 148.3738660692059, 148.45190440627334, 148.52994274334083, 148.60798108040828, 148.68601941747573, 148.76405775454322, 148.84209609161067, 148.92013442867813, 148.9981727657456, 149.07621110281306, 149.15424943988052, 149.232287776948, 149.31032611401545, 149.3883644510829, 149.4664027881504, 149.54444112521784, 149.6224794622853, 149.70051779935278, 149.77855613642024, 149.8565944734877, 149.93463281055517, 150.0126711476226, 150.09070948469008, 150.16874782175756, 150.246786158825, 150.32482449589247, 150.40286283295995, 150.48090117002738, 150.55893950709486, 150.63697784416235, 150.71501618122977, 150.79305451829725, 150.87109285536474, 150.94913119243216, 151.02716952949964, 151.1052078665671, 151.18324620363455, 151.26128454070204, 151.3393228777695, 151.41736121483694, 151.49539955190443, 151.57343788897188, 151.65147622603934, 151.72951456310682, 151.80755290017427, 151.88559123724173, 151.9636295743092, 152.04166791137666, 152.11970624844412, 152.1977445855116, 152.27578292257905, 152.3538212596465, 152.431859596714, 152.50989793378145, 152.5879362708489, 152.66597460791638, 152.7440129449838, 152.8220512820513, 152.90008961911877, 152.9781279561862, 153.05616629325368, 153.13420463032116, 153.2122429673886, 153.29028130445607, 153.36831964152356, 153.44635797859098, 153.52439631565846, 153.60243465272595, 153.68047298979337, 153.75851132686086, 153.8365496639283, 153.91458800099576, 153.99262633806325, 154.0706646751307, 154.14870301219815, 154.22674134926564, 154.3047796863331, 154.38281802340055, 154.46085636046803, 154.53889469753548, 154.61693303460294, 154.69497137167042, 154.77300970873787, 154.85104804580533, 154.9290863828728, 155.00712471994026, 155.08516305700772, 155.1632013940752, 155.24123973114266, 155.3192780682101, 155.3973164052776, 155.47535474234505, 155.5533930794125, 155.63143141647998, 155.7094697535474, 155.7875080906149, 155.86554642768237, 155.9435847647498, 156.02162310181728, 156.09966143888477, 156.1776997759522, 156.25573811301967, 156.33377645008716, 156.41181478715458, 156.48985312422207, 156.56789146128955, 156.64592979835697, 156.72396813542446, 156.80200647249194, 156.88004480955937, 156.95808314662685, 157.03612148369433, 157.11415982076176, 157.19219815782924, 157.27023649489672, 157.34827483196415, 157.42631316903163, 157.50435150609908, 157.58238984316654, 157.66042818023402, 157.73846651730148, 157.81650485436893, 157.8945431914364, 157.97258152850387, 158.05061986557132, 158.1286582026388, 158.20669653970626, 158.2847348767737, 158.3627732138412, 158.44081155090865, 158.5188498879761, 158.59688822504359, 158.67492656211104, 158.7529648991785, 158.83100323624598, 158.90904157331343, 158.98707991038088, 159.06511824744837, 159.14315658451582, 159.22119492158328, 159.29923325865076, 159.3772715957182, 159.45530993278567, 159.53334826985315, 159.61138660692058, 159.68942494398806, 159.76746328105554, 159.84550161812297, 159.92353995519045, 160.00157829225793, 160.07961662932536, 160.15765496639284, 160.23569330346032, 160.31373164052775, 160.39176997759523, 160.4698083146627, 160.54784665173014, 160.62588498879762, 160.7039233258651, 160.78196166293253]
  in  "Energy/Pixel":bool
  in  "Normalize":bool
  out "Counts at Cursor":dbl=6129.0
  in  "Substract\nBackground 3":bool
  in  "stop 4":bool
  in  "Start Measurement":bool
  in  "Number \nof Averages":i32=1
  out "Current\n Loop":i32=1
  out "Image Handle 2":u32 caption="Image Handle"
  out "XUV spectra measurement":cluster{dbl[], dbl[]}[](graph)
  in  "Save Spectrum":bool
  out "Max. Counts":dbl=11631.0
  in  "Autoscale Spectrum":bool
  in  "Save to Logbook":bool
  in  "Comment":string="0.1 sec integration time \n1200 nm Zr"
  in  "Force Camera to Close":bool
  in  "Destroy all Images":bool
  out "error out":errorcluster
  in  "error in":errorcluster
  out "Toolkit Error":bool
  in  "Parameters":T6={"camera parameters"={"Camera Handle"=16842752, "Xdim"=1340, "Ydim"=400}, "error"={"status"=FALSE, "code"=0, "source"=""}, "Plot height [pixel]"=335.0, "Plot width [pixel]"=100.0}
  out "Versions":T7={"Major Version"=4, "Minor Version"=1, "External Build"=0, "Internal Build"=2} caption="Toolkit Versions (SITK)"
  out "Number of Cameras":i32=1
  in  "Index":u32 caption="Index (Zero)"
  out "Device from ToolkitVersions":u32
  in  "Camera Index (One)":u32=1 min=1 step=1
  out "Device ID from \"GetIDs\"":u32
  out "Total Nuber of Devices or DLLs":u32=211
  out "error out":errorcluster
  in  "error in":errorcluster
  # "Binning"
  # "Integration Time [s]"
  # "Number of\n Averages"
  # "Current\n Loop"
  # "(Full Chip)"
  # "(1340)"
  # "(1)"
  # "(400)"
  # "(1)"
  # "(should be around 211)"
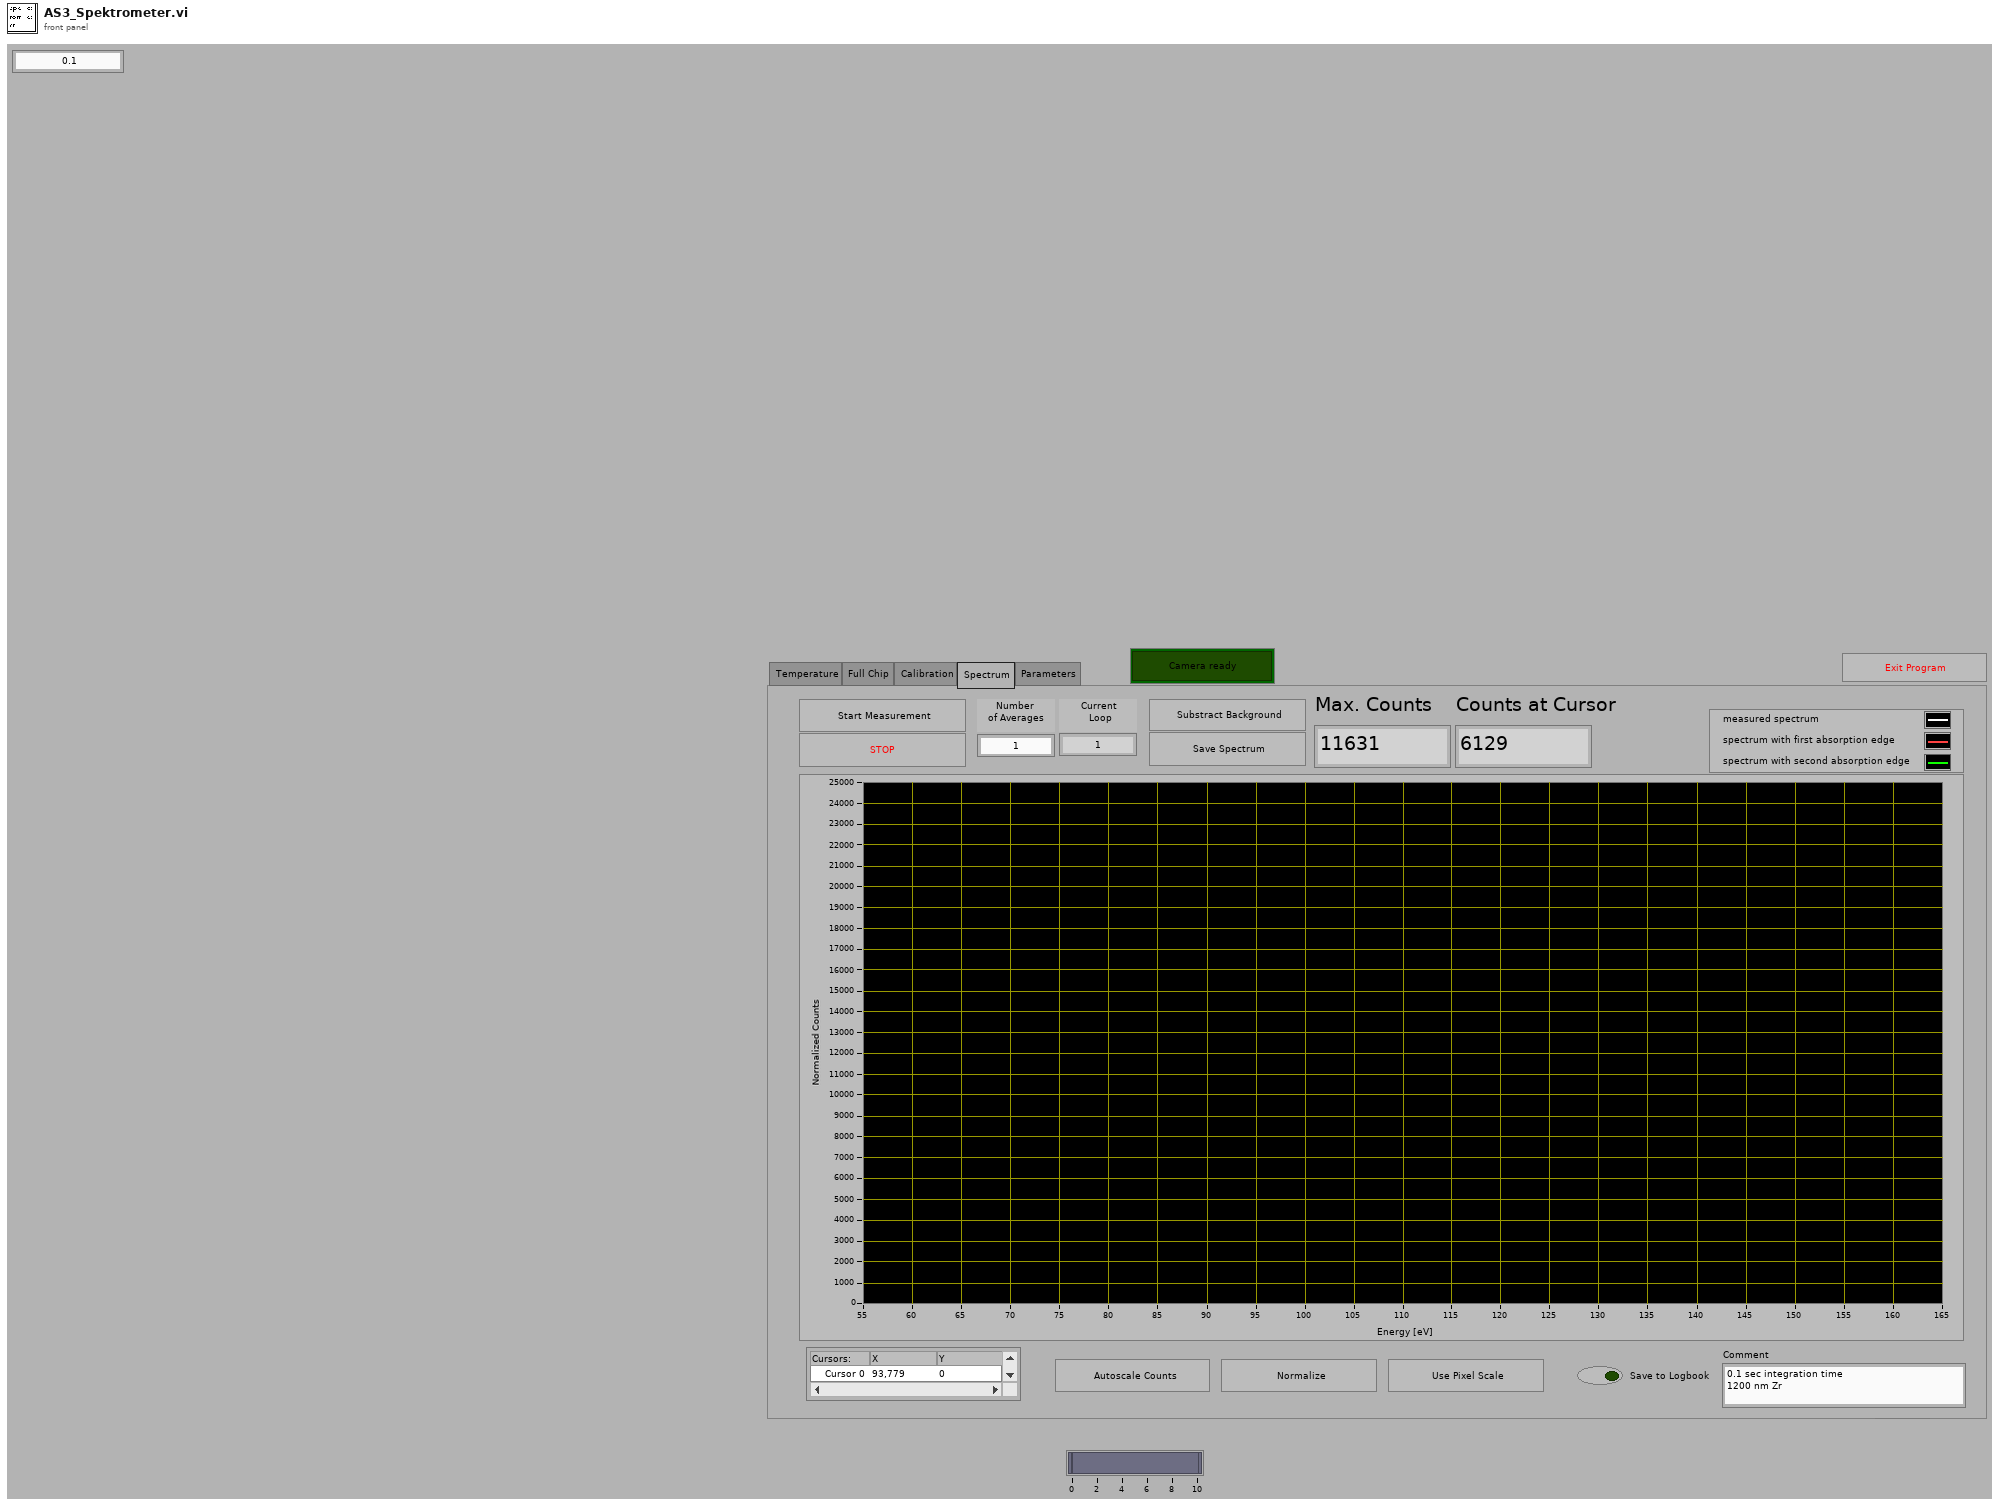
[diagram p1: front panel]
types:
  T1 = enum32{"Temperature", "Full Chip", "Calibration", "Spectrum", "Parameters"}
  T2 = cluster{"X Max":dbl, "Y Min":dbl, "X Min":dbl, "Y Max":dbl}
  T3 = cluster{"X Start":u32, "X End":u32, "Binning X":u32, "Y Start":u32, "Y End":u32, "Binning Y":u32}
  T4 = cluster{"X min":dbl, "Y min":dbl, "X max":dbl, "Y max":dbl}
  T5 = cluster{"pixel scale":dbl[], "output spectrum":dbl[]}[]
  T6 = cluster{"camera parameters":cluster{"Camera Handle":u32, "Xdim":u32, "Ydim":u32}, "error":errorcluster, "Plot height [pixel]":dbl, "Plot width [pixel]":dbl}
  T7 = cluster{"Major Version":u32, "Minor Version":u32, "External Build":u32, "Internal Build":u32}
  T8 = cluster{"X start":u32, "X end":u32, "X Binning/Grouping":u32, "Y start":u32, "Y end":u32, "Y Binning/Grouping":u32}
  T9 = cluster{"Camera Handle":u32, "Xdim":u32, "Ydim":u32}
  T10 = typedef "LVCursorListTypeDef.ctl" = cluster{"Name":string, "Color":u32, "Style":u8, "Point Style":u8, "Name Visible":bool, "Allow Drag":bool, "Cursor Mode":u32, "Plot":i32, "Index":i32, "Position":cluster{"X":dbl, "Y":dbl}, "X Scale":u32, "Y Scale":u32, "Watch Plots":i32[], "Watch All Plots":bool, "Plot Area":i32, "Label Offset":cluster{"X":dbl, "Y":dbl}}[]
  T11 = cluster{"Name":string, "Color":u32, "Style":u8, "Point Style":u8, "Name Visible":bool, "Allow Drag":bool, "Cursor Mode":u32, "Plot":i32, "Index":i32, "Position":cluster{"X":dbl, "Y":dbl}, "X Scale":u32, "Y Scale":u32, "Watch Plots":i32[], "Watch All Plots":bool, "Plot Area":i32, "Label Offset":cluster{"X":dbl, "Y":dbl}}
  T12 = cluster{"Name":string, "Color":u32, "Style":u8, "Point Style":u8, "Name Visible":bool, "Allow Drag":bool, "Cursor Mode":u32, "Plot":i32, "Index":i32, "Position":cluster{"X":dbl, "Y":dbl}, "X Scale":u32, "Y Scale":u32, "Watch Plots":i32[], "Watch All Plots":bool, "Plot Area":i32, "Label Offset":cluster{"X":dbl, "Y":dbl}}[]
  T13 = typedef "imagedata.ctl" = cluster{"image type":i32, "image depth":i32, "image":u8[], "mask":u8[], "colors":u32[], "Rectangle":cluster{"left":i16, "top":i16, "right":i16, "bottom":i16}}
  T14 = cluster{"pixel scale":dbl[], "output spectrum":dbl[]}
  T15 = cluster{"pixel scale":dbl[], "background\nspectrum":dbl[]}
  T16 = cluster{"pixel scale":dbl[], "background\nspectrum":dbl[]}[]
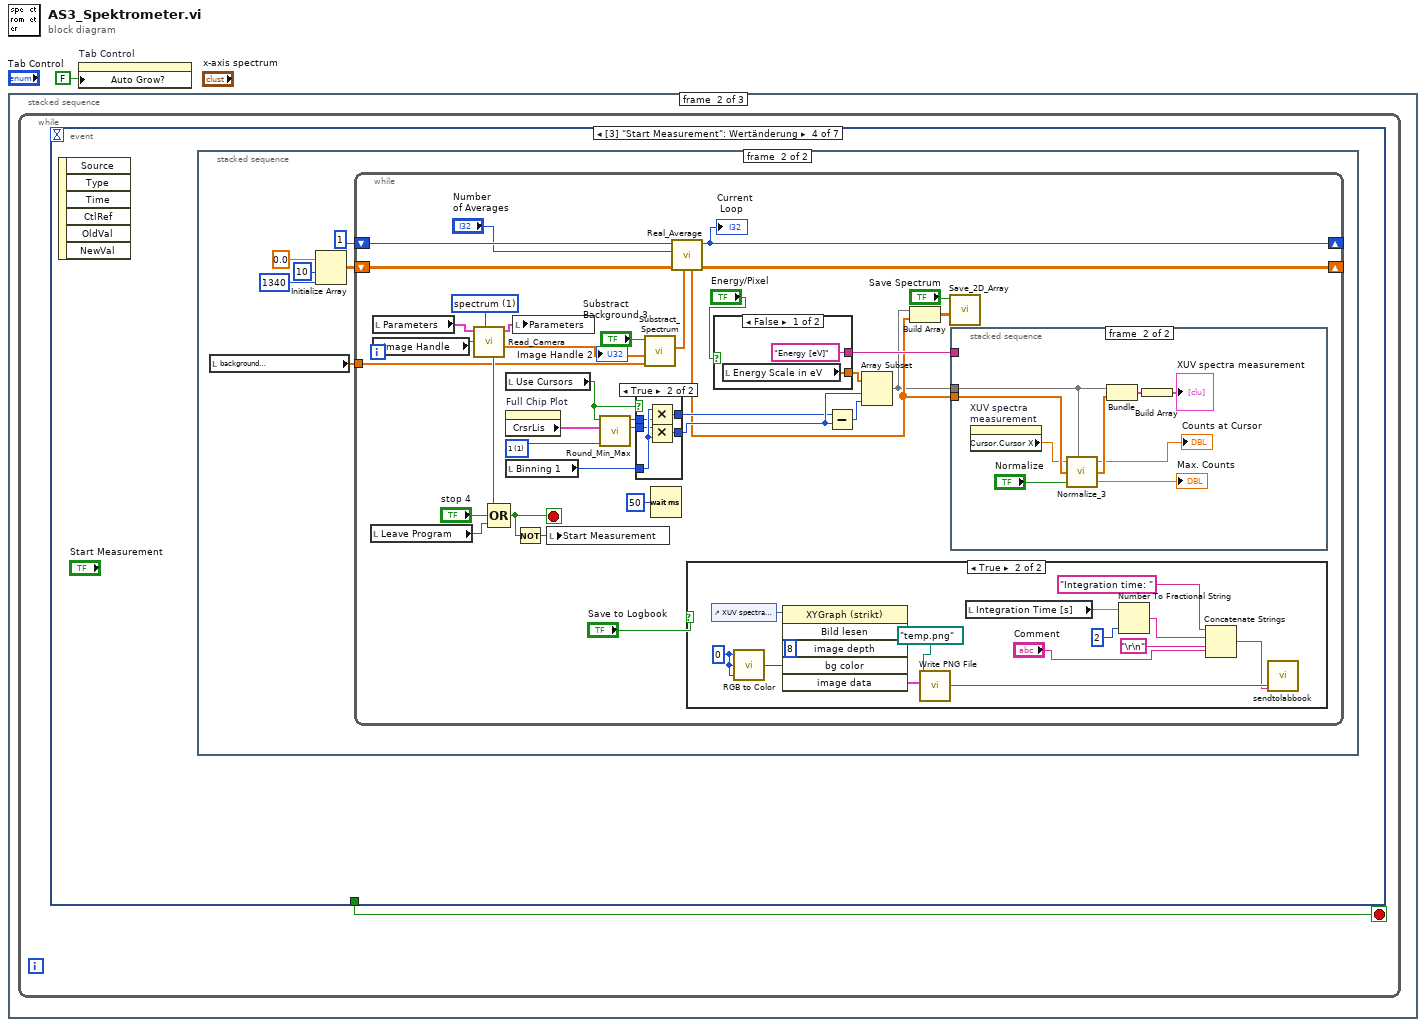
[diagram p0: block diagram]
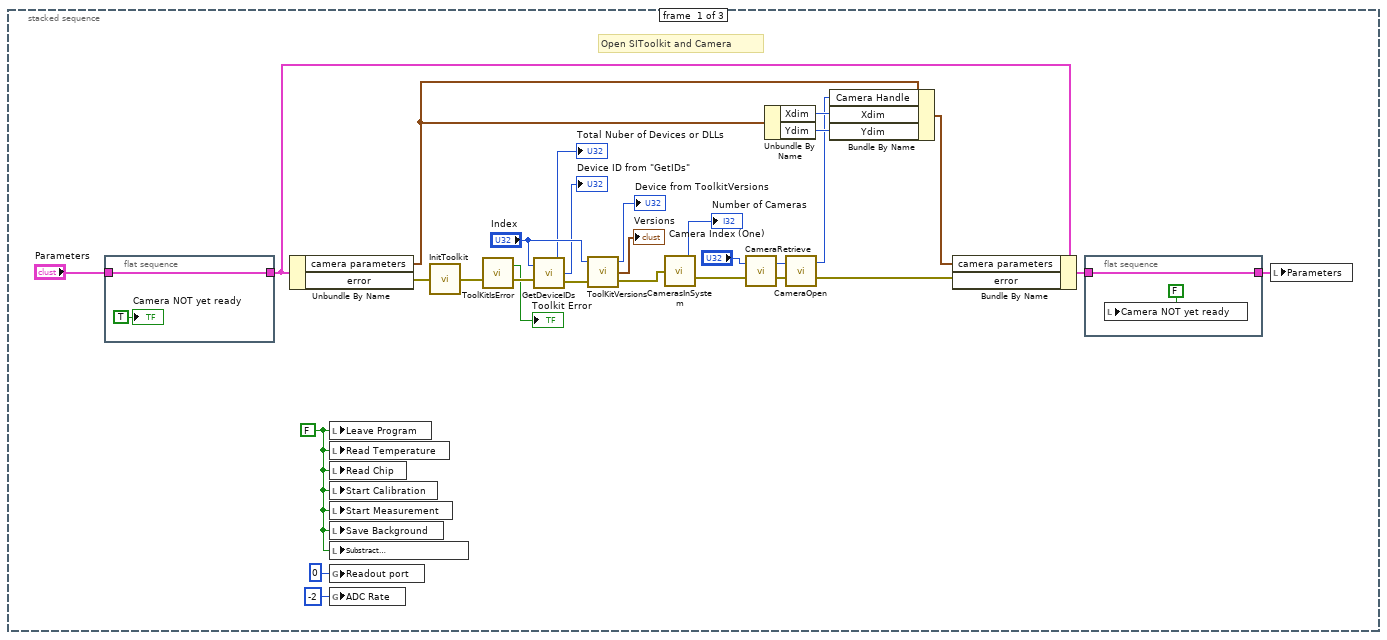
[diagram p2: hidden frame]
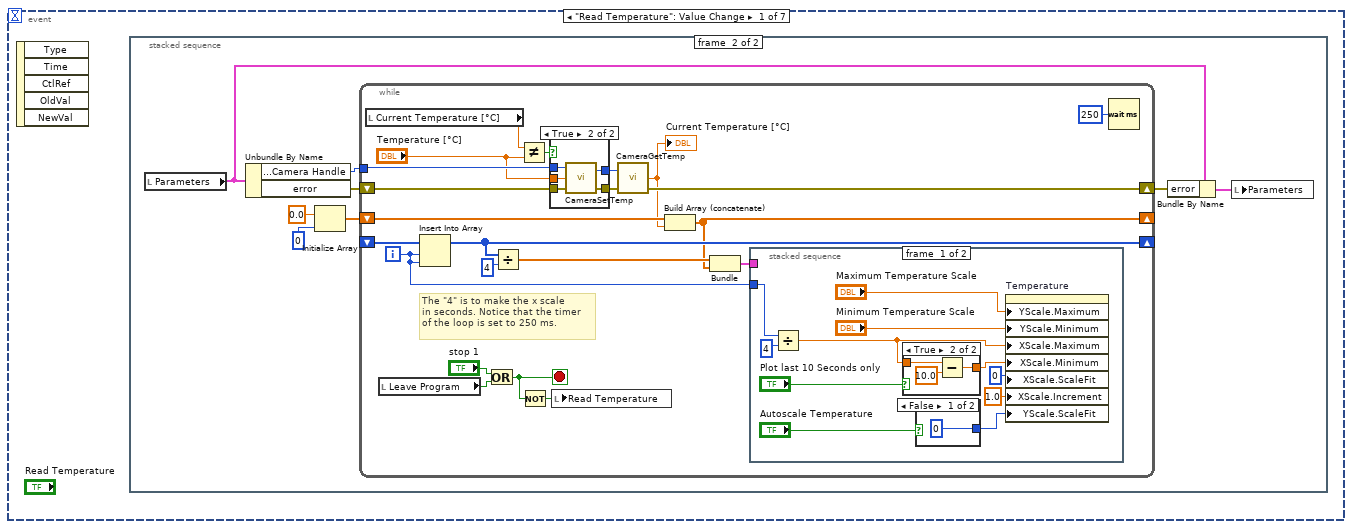
[diagram p3: hidden frame]
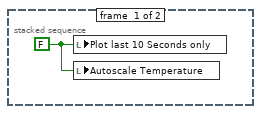
[diagram p4: hidden frame]
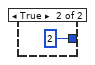
[diagram p5: hidden frame]
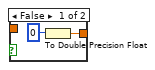
[diagram p6: hidden frame]
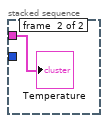
[diagram p7: hidden frame]
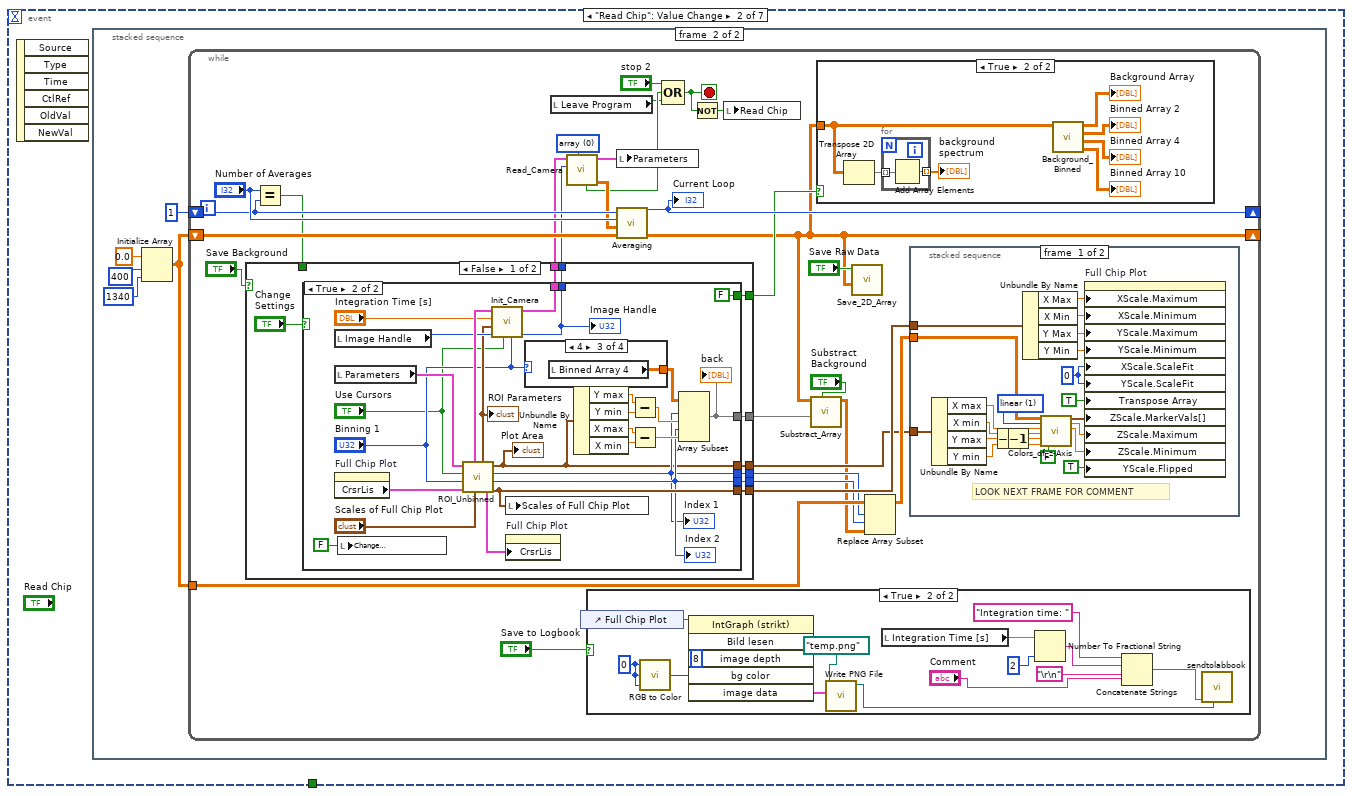
[diagram p9: hidden frame]
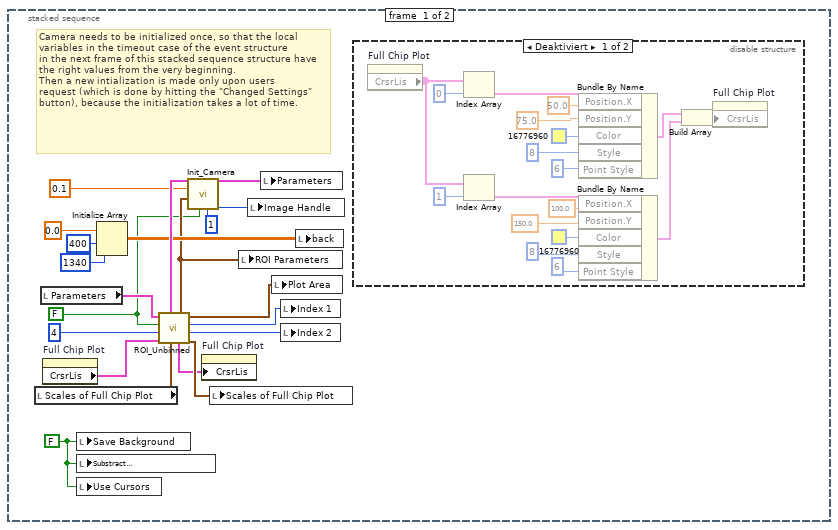
[diagram p10: hidden frame]
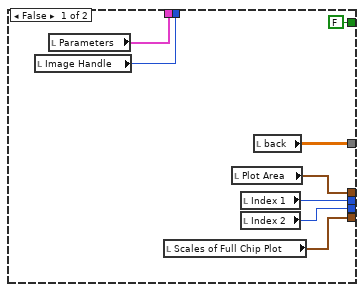
[diagram p13: hidden frame]
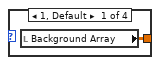
[diagram p14: hidden frame]
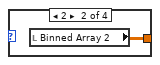
[diagram p15: hidden frame]
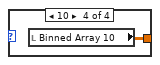
[diagram p16: hidden frame]
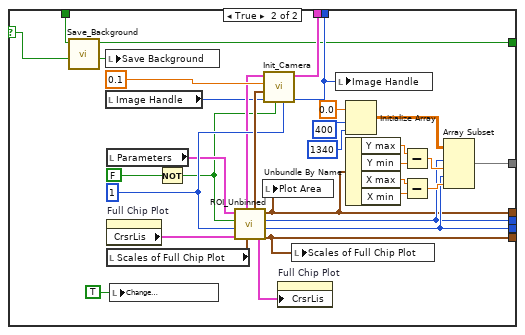
[diagram p17: hidden frame]
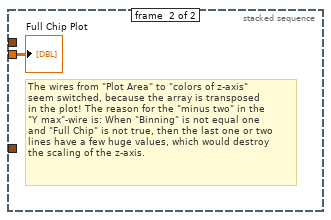
[diagram p19: hidden frame]
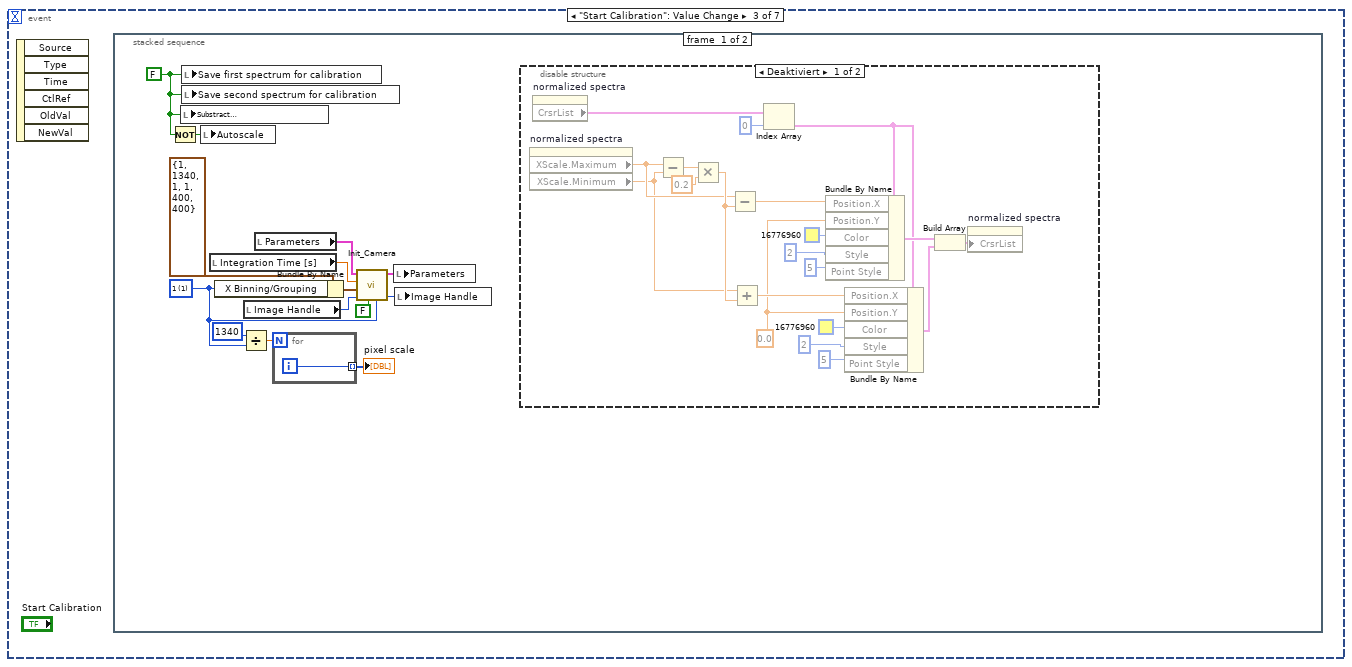
[diagram p20: hidden frame]
diagram:
  n1 = stacked-sequence {
    frame #0 {
      w2 = FALSE
      # "Open SIToolkit and Camera"
      n2 = flat-sequence {
        tunnel: "Parameters" -> [w34]
        tunnel: [w34] -> w11
        frame #0 {
          "Camera NOT yet ready" <- TRUE
        }
      }
      n3 = Unbundle By Name(w11) -> ("camera parameters"=w13:T9, "error"=w17:errorcluster)
      n4 = local write "Leave Program"(w2) -> ()
      n5 = local write "Read Temperature"(w2) -> ()
      n6 = local write "Read Chip"(w2) -> ()
      n7 = local write "Start Calibration"(w2) -> ()
      n8 = local write "Start Measurement"(w2) -> ()
      n9 = local write "Save Background"(w2) -> ()
      n10 = local write "Substract\nBackground"(w2) -> ()
      n11 = global write "readoutport.vi" "Readout port"(0) -> ()
      n12 = global write "ADC.vi" "ADC Rate"(-2) -> ()
      n13 = call <userlib>:"InitToolkit.vi"("error in"=w17) -> ("error out"=w30:errorcluster)
      n14 = call <userlib>:"ToolKitIsError.vi"("error in"=w30) -> ("error out"=w25:errorcluster, "Error Flag"=→"Toolkit Error":bool)  [unwired: 1 in]
      n15 = call <userlib>:"GetDeviceIDs.vi"("Index"="Index", "error in"=w25) -> ("Total Nuber of Devices or DLLs"=→"Total Nuber of Devices or DLLs":u32, "Device ID"=→"Device ID from \"GetIDs\"":u32, "error out"=w24:errorcluster)
      n16 = call <userlib>:"ToolKitVersions.vi"("error in"=w24, "Index"="Index") -> ("error out"=w23:errorcluster, "Versions"=→"Versions":T7, "Device"=→"Device from ToolkitVersions":u32)  [unwired: 1 in]
      n17 = call <userlib>:"CamerasInSystem.vi"("error in"=w23) -> ("Number of Cameras"=→"Number of Cameras":i32, "error out"=w27:errorcluster)
      n18 = call <userlib>:"CameraRetrieve.vi"("error in"=w27, "Camera Index"="Camera Index (One)") -> ("error out"=w29:errorcluster, "Device ID"=w28:u32)
      n19 = Unbundle By Name(w13) -> ("Xdim"=w16:u32, "Ydim"=w15:u32)
      n20 = call <userlib>:"CameraOpen.vi"("error in"=w29, "Camera Device ID"=w28) -> ("error out"=w6:errorcluster, "Camera Handle"=w5:u32)
      n21 = Bundle By Name(cluster=w13, "Camera Handle"=w5, "Xdim"=w16, "Ydim"=w15) -> (w14:T9)
      n22 = Bundle By Name(cluster=w11, "camera parameters"=w14, "error"=w6) -> (w10:T6)
      n23 = flat-sequence {
        tunnel: w10 -> [w32]
        tunnel: [w32] -> w9
        frame #0 {
          n24 = local write "Camera NOT yet ready"(FALSE) -> ()
        }
      }
      n25 = local write "Parameters"(w9) -> ()
    }
    frame #1 {
      n26 = while {
        stop <- w35 stop-if-true
        n27 = event shown="[3] \"Start Measurement\": Wertänderung" {
          selector: _ -> [_ _ _ _ _ _ _]
          dyn-events: _ -> [_ _ _ _ _ _ _]
          timeout: _ -> [_ _ _ _ _ _ _]
          tunnel: [_ _ _ _ _ _ "Leave Program"] -> w35
          event "Read Temperature": Value Change {
            n28 = event-data() -> ()  [unwired: 1 in, 5 out]
            n29 = stacked-sequence {
              frame #0 {
                w36 = FALSE ("Read Temperature")
                n30 = local write "Plot last 10 Seconds only"(w36) -> ()
                n31 = local write "Autoscale Temperature"(w36) -> ()
              }
              frame #1 {
                n32 = local read "Parameters"() -> (w40:T6)
                n33 = Unbundle By Name(w40) -> ("camera parameters.Camera Handle"=w43:u32, "error"=w42:errorcluster)
                n34 = Initialize Array(0.0 ("element"), 0 ("dimension size")) -> (w37:dbl[])
                n35 = while {
                  tunnel: w43 -> [w66]
                  shift-right: [w63] -> w44
                  shift-left: w42 -> [w62]
                  shift-right: [w50] -> _
                  shift-left: w37 -> [w49]
                  shift-right: [w54] -> _
                  shift-left: _ -> [w55]
                  i -> [w48]
                  stop <- w46 stop-if-true
                  # "The \"4\" is to make the x scale\nin seconds. Notice that the timer\nof the loop is set to 250 ms."
                  n36 = local read "Current Temperature [°C]"() -> (w58:dbl)
                  n37 = local read "Leave Program"() -> (w56:bool)
                  n38 = Insert Into Array(array=w55, index=w48, new element=w48) -> (w54:i32[])
                  n39 = Or(x="stop 1", y=w56) -> (x .or. y?=w46:bool)
                  n40 = Divide(x=w54, y=4) -> (x/y=w52:dbl[])
                  n41 = Not Equal?(x=w58, y="Temperature [°C]") -> (x != y?=w61:bool)
                  n42 = Not(x=w46) -> (.not. x?=w45:bool)
                  n43 = case shown="True" w61 {
                    tunnel: w66 -> [w87 w92]
                    tunnel: w62 -> [w86 w91]
                    tunnel: "Temperature [°C]" -> [_ w88]
                    tunnel: [w86 w90] -> w65
                    tunnel: [w87 w89] -> w64
                    frame False {
                    }
                    frame True {
                      n44 = call <userlib>:"CameraSetTemp.vi"("error in (no error)"=w91, "Temperature"=w88, "Camera Handle"=w92) -> ("error out"=w90:errorcluster, "Camera Handle"=w89:u32)
                    }
                  }
                  n45 = local write "Read Temperature"(w45) -> ()
                  n46 = call <userlib>:"CameraGetTemp.vi"("Camera Handle"=w64, "error in (no error)"=w65) -> ("Temperature"=w47:dbl, "error out"=w63:errorcluster)  [unwired: 1 out]
                  "Current Temperature [°C]" <- w47
                  n47 = Build Array (concatenate)(w49, w47) -> (w50:dbl[])
                  n48 = Bundle(w52, w50) -> (w51:cluster{dbl[], dbl[]})  [unwired: 1 in]
                  n49 = stacked-sequence {
                    tunnel: w51 -> [_ w85]
                    tunnel: w48 -> [w73 _]
                    frame #0 {
                      n50 = Divide(x=w73, y=4) -> (x/y=w67:dbl)
                      n51 = case shown="True" "Plot last 10 Seconds only" {
                        tunnel: w67 -> [_ w82]
                        tunnel: [w80 w84] -> w74
                        frame False {
                          n52 = To Double Precision Float(number=0) -> (double precision float=w80:dbl)
                        }
                        frame True {
                          n53 = Subtract(x=w82, y=10.0) -> (x-y=w84:dbl)
                        }
                      }
                      n54 = case shown="False" "Autoscale Temperature" {
                        tunnel: [u8 0 ("Y Scale.Scale Fit") u8 2 ("Y Scale.Scale Fit")] -> w68
                        frame False {
                        }
                        frame True {
                        }
                      }
                      n55 = property on="Temperature" class="XYGraph (strikt)"("YScale.Maximum"="Maximum Temperature Scale", "YScale.Minimum"="Minimum Temperature Scale", "XScale.Maximum"=w67, "XScale.Minimum"=w74, "XScale.ScaleFit"=u8 0 ("Y Scale.Scale Fit"), "XScale.Increment"=1.0 ("X Scale.Range:Minor Increment"), "YScale.ScaleFit"=w68) -> ()  [unwired: 2 in, 2 out]
                    }
                    frame #1 {
                      "Temperature" <- w85
                    }
                  }
                  n56 = Wait (ms)(milliseconds to wait=u32 250 ("Zu wartende ms")) -> ()  [unwired: 1 out]
                }
                n57 = Bundle By Name(cluster=w40, "error"=w44) -> (w41:T6)
                n58 = local write "Parameters"(w41) -> ()
              }
            }
          }
          event "Read Chip": Value Change {
            n59 = event-data() -> ()  [unwired: 1 in, 6 out]
            n60 = stacked-sequence {
              frame #0 {
                w93 = FALSE ("Full Chip")
                w95 = FALSE ("Save Background")
                # "Camera needs to be initialized once, so that the local\nvariables in the timeout case of the event structure\nin the next frame of this stacked sequence structure have the right values from the very beginning.\nThen a new intialization is made only upon users \nrequest (which is done by hitting the \"Changed Settings\"\nbutton), because the initialization takes a lot of time."
                n61 = local read "Scales of Full Chip Plot"() -> (w100:T2)
                n62 = local read "Parameters"() -> (w112:T6)
                n63 = property on="Full Chip Plot" class="IntGraph (strikt)"() -> ("CrsrLis"=w99:T10)  [unwired: 2 in, 2 out]
                n64 = local write "Save Background"(w95) -> ()
                n65 = local write "Substract\nBackground"(w95) -> ()
                n66 = local write "Use Cursors"(w95) -> ()
                n67 = Initialize Array(0.0 ("element"), 400 ("dimension size"), 1340 ("dimension size")) -> (w101:dbl[][])
                n68 = call "ROI_Unbinned.vi"("Scales IN"=w100, "CrsList"=w99, "Binning"=u32 4, "Use Cursors"=w93, "Parameters IN"=w112) -> ("Scales of Full Chip Plot"=w107:T2, "Index 2"=w108:u32, "Index 1"=w109:u32, "Plot Area"=w110:T4, "CrsList OUT"=w98:T10, "ROI Parameters"=w97:T3, "Parameters OUT"=w113:T6)
                n69 = call "Init_Camera.vi"("Binning IN"=u32 1 ("Binning"), "Use Cursors IN"=w93, "ROI Parameters"=w97, "integration time [s]"=0.1 ("Integration Time [s]"), "Parameters IN"=w113) -> ("Image Handle OUT"=w96:u32, "Parameters OUT"=w111:T6)  [unwired: 5 in]
                n70 = property on="Full Chip Plot" class="IntGraph (strikt)"("CrsrLis"=w98) -> ()  [unwired: 2 in, 2 out]
                n71 = local write "Scales of Full Chip Plot"(w107) -> ()
                n72 = local write "ROI Parameters"(w97) -> ()
                n73 = local write "Image Handle"(w96) -> ()
                n74 = local write "Parameters"(w111) -> ()
                n75 = local write "Plot Area"(w110) -> ()
                n76 = local write "Index 1"(w109) -> ()
                n77 = local write "Index 2"(w108) -> ()
                n78 = local write "back"(w101) -> ()
                n79 = disable-structure shown="Deaktiviert" {
                  frame Disabled {
                    n80 = property on="Full Chip Plot" class="IntGraph (strikt)"() -> ("CrsrLis"=w125:T10)  [unwired: 2 in, 2 out]
                    n81 = Index Array(array=w125, index=0) -> (element=w127:T11)
                    n82 = Index Array(array=w125, index=1) -> (element=w126:T11)
                    n83 = Bundle By Name(cluster=w127, "Position.X"=50.0, "Position.Y"=75.0, "Color"=u32 16776960, "Style"=u8 8, "Point Style"=u8 6) -> (w131:T11)
                    n84 = Bundle By Name(cluster=w126, "Position.X"=100.0, "Position.Y"=150.0, "Color"=u32 16776960, "Style"=u8 8, "Point Style"=u8 6) -> (w130:T11)
                    n85 = Build Array(w131, w130) -> (w120:T12)
                    n86 = property on="Full Chip Plot" class="IntGraph (strikt)"("CrsrLis"=w120) -> ()  [unwired: 2 in, 2 out]
                  }
                  frame Enabled {
                  }
                }
              }
              frame #1 {
                n87 = Initialize Array(0.0 ("element"), 400 ("dimension size"), 1340 ("dimension size")) -> (w132:dbl[][])
                n88 = while {
                  shift-right: [w162] -> _
                  shift-left: 1 ("next measurement number") -> [w160]
                  tunnel: w132 -> [w163]
                  shift-right: [w138] -> _
                  shift-left: w132 -> [w164]
                  stop <- w159 stop-if-true
                  w151 = u16 0 items=["array", "spectrum"] ("data type")
                  n89 = Equal?(x="Number of Averages", y=w160) -> (x = y?=w140:bool)
                  n90 = case shown="False" "Save Background" {
                    selector: "Save Background" -> [_ w230]
                    tunnel: [w188 w241] -> w156
                    tunnel: [w187 w240] -> w155
                    tunnel: [w186 w239] -> w154
                    tunnel: [w185 w235] -> w153
                    tunnel: [w184 w232] -> w152
                    tunnel: [w182 w231] -> w150
                    tunnel: [w181 w233] -> w144
                    tunnel: w140 -> [_ w229]
                    tunnel: [w180 w227] -> w139
                    frame False {
                      n91 = case shown="True" "Change\nSettings" {
                        tunnel: [w194 w206] -> w188
                        tunnel: [w195 w205] -> w187
                        tunnel: [w196 w204] -> w186
                        tunnel: [w193 w203] -> w185
                        tunnel: [w191 w202] -> w184
                        tunnel: [w190 w201] -> w182
                        tunnel: [w192 w200] -> w181
                        tunnel: [FALSE FALSE] -> w180
                        frame False {
                          n92 = local read "Image Handle"() -> (w191:u32)
                          n93 = local read "Parameters"() -> (w190:T6)
                          n94 = local read "Scales of Full Chip Plot"() -> (w194:T2)
                          n95 = local read "Plot Area"() -> (w193:T4)
                          n96 = local read "Index 1"() -> (w196:u32)
                          n97 = local read "Index 2"() -> (w195:u32)
                          n98 = local read "back"() -> (w192:dbl[][])
                        }
                        frame True {
                          n99 = local read "Image Handle"() -> (w209:u32)
                          n100 = local read "Parameters"() -> (w212:T6)
                          n101 = property on="Full Chip Plot" class="IntGraph (strikt)"() -> ("CrsrLis"=w213:T10)  [unwired: 2 in, 2 out]
                          n102 = local write "Change\nSettings"(FALSE ("Settings Changed")) -> ()
                          n103 = call "ROI_Unbinned.vi"("Scales IN"="Scales of Full Chip Plot", "CrsList"=w213, "Binning"="Binning 1", "Use Cursors"="Use Cursors", "Parameters IN"=w212) -> ("Scales of Full Chip Plot"=w206:T2, "Index 2"=w205:u32, "Index 1"=w204:u32, "Plot Area"=w203:T4, "CrsList OUT"=w215:T10, "ROI Parameters"=w208:T3, "Parameters OUT"=w211:T6)
                          "ROI Parameters" <- w208
                          "Plot Area" <- w203
                          "Index 1" <- w204
                          "Index 2" <- w205
                          n104 = call "Init_Camera.vi"("Binning IN"="Binning 1", "Use Cursors IN"="Use Cursors", "Image Handle IN"=w209, "ROI Parameters"=w208, "integration time [s]"="Integration Time [s]", "Parameters IN"=w211) -> ("Image Handle OUT"=w202:u32, "Parameters OUT"=w201:T6)  [unwired: 4 in]
                          "Image Handle" <- w202
                          n105 = local write "Scales of Full Chip Plot"(w206) -> ()
                          n106 = property on="Full Chip Plot" class="IntGraph (strikt)"("CrsrLis"=w215) -> ()  [unwired: 2 in, 2 out]
                          n107 = case shown="4" "Binning 1" {
                            tunnel: [w223 w224 w225 w226] -> w216
                            frame 1, Default {
                              n108 = local read "Background Array"() -> (w223:dbl[][])
                            }
                            frame 2 {
                              n109 = local read "Binned Array 2"() -> (w224:dbl[][])
                            }
                            frame 4 {
                              n110 = local read "Binned Array 4"() -> (w225:dbl[][])
                            }
                            frame 10 {
                              n111 = local read "Binned Array 10"() -> (w226:dbl[][])
                            }
                          }
                          n112 = Unbundle By Name(w203) -> ("Y max"=w220:dbl, "Y min"=w219:dbl, "X max"=w218:dbl, "X min"=w217:dbl)
                          n113 = Subtract(x=w220, y=w219) -> (x-y=w222:dbl)
                          n114 = Subtract(x=w218, y=w217) -> (x-y=w221:dbl)
                          n115 = Array Subset(array=w216, index (row)=w204, length (row)=w222, index (col)=w205, length (col)=w221) -> (w200:dbl[][])
                          "back" <- w200
                        }
                      }
                    }
                    frame True {
                      w257 = u32 1 ("Binning")
                      n116 = call "Save_Background.vi"("button"=w230, "averaging complete"=w229) -> ("button on"=w228:bool, "save spectrum"=w227:bool)  [unwired: 8 in]
                      n117 = local write "Save Background"(w228) -> ()
                      n118 = local read "Image Handle"() -> (w244:u32)
                      n119 = local read "Parameters"() -> (w246:T6)
                      n120 = property on="Full Chip Plot" class="IntGraph (strikt)"() -> ("CrsrLis"=w247:T10)  [unwired: 2 in, 2 out]
                      n121 = local read "Scales of Full Chip Plot"() -> (w259:T2)
                      n122 = local write "Change\nSettings"(TRUE ("Settings Changed")) -> ()
                      n123 = Not(x=FALSE ("Settings Changed")) -> (.not. x?=w242:bool)
                      n124 = call "ROI_Unbinned.vi"("Scales IN"=w259, "CrsList"=w247, "Binning"=w257, "Use Cursors"=w242, "Parameters IN"=w246) -> ("Scales of Full Chip Plot"=w241:T2, "Index 2"=w240:u32, "Index 1"=w239:u32, "Plot Area"=w235:T4, "CrsList OUT"=w248:T10, "ROI Parameters"=w258:T3, "Parameters OUT"=w245:T6)
                      n125 = local write "Plot Area"(w235) -> ()
                      n126 = call "Init_Camera.vi"("Binning IN"=w257, "Use Cursors IN"=w242, "Image Handle IN"=w244, "ROI Parameters"=w258, "integration time [s]"=0.1, "Parameters IN"=w245) -> ("Image Handle OUT"=w232:u32, "Parameters OUT"=w231:T6)  [unwired: 4 in]
                      n127 = property on="Full Chip Plot" class="IntGraph (strikt)"("CrsrLis"=w248) -> ()  [unwired: 2 in, 2 out]
                      n128 = local write "Scales of Full Chip Plot"(w241) -> ()
                      n129 = local write "Image Handle"(w232) -> ()
                      n130 = Initialize Array(0.0 ("element"), 400 ("dimension size"), 1340 ("dimension size")) -> (w234:dbl[][])
                      n131 = Unbundle By Name(w235) -> ("Y max"=w252:dbl, "Y min"=w251:dbl, "X max"=w250:dbl, "X min"=w249:dbl)
                      n132 = Subtract(x=w252, y=w251) -> (x-y=w254:dbl)
                      n133 = Subtract(x=w250, y=w249) -> (x-y=w253:dbl)
                      n134 = Array Subset(array=w234, index (row)=w239, length (row)=w254, index (col)=w240, length (col)=w253) -> (w233:dbl[][])
                    }
                  }
                  n135 = local read "Leave Program"() -> (w145:bool)
                  n136 = call "Read_Camera.vi"("data type"=w151, "Image Handle IN"=w152, "input parameters"=w150) -> ("array"=w157:dbl[][], "output parameters"=w149:T6, "exit program"=w146:bool)  [unwired: 4 in, 2 out]
                  n137 = case shown="True" "Save to Logbook" {
                    frame False {
                    }
                    frame True {
                      w177 = u8 0 ("R")
                      n138 = control-ref of="Full Chip Plot"() -> (w173:refnum<vi>)
                      n139 = call <vilib>:"RGB to Color.vi"("B"=w177, "G"=w177, "R"=w177) -> ("Color"=w178:u32)
                      n140 = invoke on="Methodenknoten" class="IntGraph (strikt)" method="Bild lesen"(reference=w173, "image depth"=8 ("Image Depth"), "bg color"=w178) -> ("image data"=w179:T13)  [unwired: 3 in, 5 out]
                      n141 = call <vilib>:"Write PNG File.vi"("image data"=w179, "path to PNG file"=path "temp.png") -> ("path"=w174:path)  [unwired: 8 in, 1 out]
                      n142 = local read "Integration Time [s]"() -> (w169:dbl)
                      n143 = Number To Fractional String(number=w169, precision (6)=2) -> (F-format string=w170:string)  [unwired: 2 in]
                      n144 = Concatenate Strings("Integration time: " ("String"), w170, "\r\n", "Comment") -> (w168:string)
                      n145 = call "sendtolabbook.vi"("File"=w174, "Text"=w168) -> ()  [unwired: 9 in, 1 out]
                    }
                  }
                  n146 = local write "Parameters"(w149) -> ()
                  n147 = call "Averaging.vi"("old input array"=w164, "new input array"=w157, "Number of averages"="Number of Averages", "current measurement number"=w160) -> ("output array"=w138:dbl[][], "next measurement number"=w162:i32)  [unwired: 6 in]
                  "Current Loop" <- w162
                  n148 = Compound Arithmetic op=OR("stop 2", w146, w145) -> (w159:bool)
                  n149 = Not(x=w159) -> (.not. x?=w148:bool)
                  n150 = local write "Read Chip"(w148) -> ()
                  n151 = call "Substract_Array.vi"("Substract Background"="Substract\nBackground", "Background"=w144, "Array"=w138) -> ("Output Array"=w143:dbl[][])  [unwired: 8 in]
                  n152 = case shown="True" w139 {
                    tunnel: w138 -> [_ w260]
                    frame False {
                    }
                    frame True {
                      n153 = Transpose 2D Array(2D array=w260) -> (transposed array=w265:dbl[][])
                      n154 = for {
                        tunnel: w265 -> [w268] mode=indexing
                        tunnel: [w267] -> w266 mode=indexing
                        n155 = Add Array Elements(numeric array=w268) -> (sum=w267:dbl)
                      }
                      "background\nspectrum" <- w266
                      n156 = call "Background_Binned.vi"("Background Array"=w260) -> ("Binned Array 10"=→"Binned Array 10":dbl[][], "Binned Array 4"=→"Binned Array 4":dbl[][], "Binned Array 2"=→"Binned Array 2":dbl[][], "Binned Array 1"=→"Background Array":dbl[][])  [unwired: 7 in]
                    }
                  }
                  n157 = call "Save_2D_Array.vi"("Array"=w138, "Save"="Save Raw Data") -> ()  [unwired: 10 in]
                  n158 = Replace Array Subset(array=w163, new element=w143, index (row)=w154, index (col)=w155) -> (w158:dbl[][])
                  n159 = stacked-sequence {
                    tunnel: w158 -> [w287 w290]
                    tunnel: w156 -> [w271 _]
                    tunnel: w153 -> [w272 _]
                    frame #0 {
                      w284 = u16 1 items=["logarithmic", "linear"] ("scaling")
                      w289 = 0 ("next measurement number")
                      # "LOOK NEXT FRAME FOR COMMENT"
                      n160 = Unbundle By Name(w272) -> ("X max"=w282:dbl, "X min"=w281:dbl, "Y max"=w279:dbl, "Y min"=w283:dbl)
                      n161 = Decrement(x=w279) -> (x-1=w278:dbl)
                      n162 = Decrement(x=w278) -> (x-1=w280:dbl)
                      n163 = Unbundle By Name(w271) -> ("X Max"=w270:dbl, "X Min"=w269:dbl, "Y Max"=w274:dbl, "Y Min"=w273:dbl)
                      n164 = call "Colors_of_z-Axis.vi"("Array"=w287, "scaling"=w284, "Y Scale.Range:Maximum"=w282, "Y Scale.Range:Minimum"=w281, "X Scale.Range:Maximum"=w280, "X Scale.Range:Minimum"=w283, "complete array"=FALSE) -> ("Colors"=w277:cluster{dbl, u32}[], "Maximum"=w276:dbl, "Minimum"=w275:dbl)  [unwired: 10 in]
                      n165 = property on="Full Chip Plot" class="IntGraph (strikt)"("XScale.Maximum"=w270, "XScale.Minimum"=w269, "YScale.Maximum"=w274, "YScale.Minimum"=w273, "XScale.ScaleFit"=w289, "YScale.ScaleFit"=w289, "Transpose Array"=TRUE, "ZScale.MarkerVals[]"=w277, "ZScale.Maximum"=w276, "ZScale.Minimum"=w275, "YScale.Flipped"=TRUE ("Y Scale.Flipped")) -> ()  [unwired: 2 in, 2 out]
                    }
                    frame #1 {
                      # "The wires from \"Plot Area\" to \"colors of z-axis\" \nseem switched, because the array is transposed\nin the plot! The reason for the \"minus two\" in the\n\"Y max\"-wire is: When \"Binning\" is not equal one\nand \"Full Chip\" is not true, then the last one or two\nlines have a few huge values, which would destroy\nthe scaling of the z-axis."
                      "Full Chip Plot" <- w290
                    }
                  }
                }
              }
            }
          }
          event "Start Calibration": Value Change {
            n166 = event-data() -> ()  [unwired: 1 in, 6 out]
            n167 = stacked-sequence {
              frame #0 {
                w291 = u32 1 items=["1"=1, "2"=2, "4"=4, "10"=10] ("Binning 1")
                w303 = FALSE ("Substract Background 2")
                n168 = Not(x=w303) -> (.not. x?=w304:bool)
                n169 = local write "Substract\nBackground 2"(w303) -> ()
                n170 = local write "Save first spectrum for calibration"(w303) -> ()
                n171 = local write "Save second spectrum for calibration"(w303) -> ()
                n172 = local write "Autoscale"(w304) -> ()
                n173 = local read "Integration Time [s]"() -> (w302:dbl)
                n174 = Bundle By Name(cluster=T8 {"X start"=1, "X end"=1340, "X Binning/Grouping"=1, "Y start"=1, "Y end"=400, "Y Binning/Grouping"=400} ("ROI Parameters"), "X Binning/Grouping"=w291) -> (w295:T8)
                n175 = Divide(x=u32 1340, y=w291) -> (x/y=w293:dbl)
                n176 = local read "Image Handle"() -> (w298:u32)
                n177 = local read "Parameters"() -> (w301:T6)
                n178 = for {
                  N: w293 -> [_]
                  tunnel: [w305] -> w292 mode=indexing
                  i -> [w305]
                }
                "pixel scale" <- w292
                n179 = call "Init_Camera.vi"("Binning IN"=w291, "Use Cursors IN"=FALSE ("Full Chip IN"), "Image Handle IN"=w298, "ROI Parameters"=w295, "integration time [s]"=w302, "Parameters IN"=w301) -> ("Image Handle OUT"=w299:u32, "Parameters OUT"=w300:T6)  [unwired: 4 in]
                n180 = local write "Parameters"(w300) -> ()
                n181 = local write "Image Handle"(w299) -> ()
                n182 = disable-structure shown="Deaktiviert" {
                  frame Disabled {
                    w317 = 0.0 ("Position.Y")
                    n183 = property on="normalized spectra" class="XYGraph (strikt)"() -> ("XScale.Maximum"=w308:dbl, "XScale.Minimum"=w307:dbl)  [unwired: 2 in, 2 out]
                    n184 = property on="normalized spectra" class="XYGraph (strikt)"() -> ("CrsrList"=w310:T10)  [unwired: 2 in, 2 out]
                    n185 = Subtract(x=w308, y=w307) -> (x-y=w323:dbl)
                    n186 = Multiply(x=w323, y=0.2) -> (x*y=w321:dbl)
                    n187 = Subtract(x=w308, y=w321) -> (x-y=w320:dbl)
                    n188 = Add(x=w307, y=w321) -> (x+y=w319:dbl)
                    n189 = Index Array(array=w310, index=0) -> (element=w309:T11)
                    n190 = Bundle By Name(cluster=w309, "Position.X"=w320, "Position.Y"=w317, "Color"=u32 16776960, "Style"=u8 2, "Point Style"=u8 5) -> (w325:T11)
                    n191 = Bundle By Name(cluster=w309, "Position.X"=w319, "Position.Y"=w317, "Color"=u32 16776960, "Style"=u8 2, "Point Style"=u8 5) -> (w324:T11)
                    n192 = Build Array(w325, w324) -> (w306:T12)
                    n193 = property on="normalized spectra" class="XYGraph (strikt)"("CrsrList"=w306) -> ()  [unwired: 2 in, 2 out]
                  }
                  frame Enabled {
                  }
                }
              }
              frame #1 {
                n194 = local read "background\nspectrum"() -> (w333:dbl[])
                n195 = local read "normalized spectra"() -> (w331:cluster{dbl[], dbl[]}[])
                n196 = local read "Energy Scale in eV"() -> (w330:dbl[])
                n197 = local read "pixel scale"() -> (w332:dbl[])
                n198 = Initialize Array(0.0 ("element"), 10 ("Dimension"), 1340 ("dimension size")) -> (w329:dbl[][])
                n199 = while {
                  shift-right: [w364] -> _
                  shift-left: w331 -> [w368]
                  shift-right: [w336] -> _
                  shift-left: 1 -> [w341]
                  tunnel: w333 -> [w343]
                  tunnel: w332 -> [w351]
                  shift-right: [w345] -> _
                  shift-left: w330 -> [w346]
                  shift-right: [w335] -> _
                  shift-left: w329 -> [w339]
                  stop <- w366 stop-if-true
                  w356 = u16 1 items=["array", "spectrum"] ("average")
                  n200 = local read "Image Handle"() -> (w365:u32)
                  n201 = local read "Leave Program"() -> (w384:bool)
                  n202 = local read "Parameters"() -> (w367:T6)
                  n203 = Equal?(x="Number of\nAverages", y=w341) -> (x = y?=w376:bool)
                  n204 = call "Save_Spectrum.vi"("button on"="Save second spectrum for calibration", "averaging complete"=w376) -> ("button on"=w377:bool, "save spectrum"=w374:bool)
                  n205 = call "Save_Spectrum.vi"("button on"="Save first spectrum for calibration", "averaging complete"=w376) -> ("button on"=w378:bool, "save spectrum"=w375:bool)
                  n206 = call "Read_Camera.vi"("data type"=w356, "Image Handle IN"=w365, "input parameters"=w367) -> ("spectrum"=w344:dbl[], "output parameters"=w381:T6, "exit program"=w358:bool)  [unwired: 4 in, 2 out]
                  n207 = local write "Save second spectrum for calibration"(w377) -> ()
                  n208 = local write "Save first spectrum for calibration"(w378) -> ()
                  n209 = Compound Arithmetic op=OR(w358, "stop 3", w384) -> (w366:bool)
                  n210 = local write "Parameters"(w381) -> ()
                  n211 = Not(x=w366) -> (.not. x?=w355:bool)
                  n212 = call "Substract_Spectrum.vi"("Substract Background"="Substract\nBackground 2", "spectrum"=w344, "background spectrum"=w343) -> ("output spectrum"=w338:dbl[])  [unwired: 7 in]
                  n213 = local write "Start Calibration"(w355) -> ()
                  n214 = call "Real_Average.vi"("new input spectrum"=w338, "old input array"=w339, "Number of averages"="Number of\nAverages", "current measurement number"=w341) -> ("output array"=w335:dbl[][], "next measurement number"=w336:i32, "output spectrum"=w337:dbl[])  [unwired: 5 in]
                  "Current\nLoop" <- w336
                  n215 = call "Normalize_3.vi"("raw data"=w337, "Normalize"=TRUE) -> ("raw data"=w353:dbl[])  [unwired: 5 in, 2 out]
                  n216 = Bundle("pixel scale"=w351, "raw data"=w353) -> (w361:cluster{"pixel scale":dbl[], "raw data":dbl[]})  [unwired: 1 in]
                  n217 = Or(x=w375, y=w374) -> (x .or. y?=w369:bool)
                  n218 = Build Array(FALSE ("element"), w375, w374) -> (w372:bool[])
                  n219 = Boolean To (0,1)(Boolean=w372) -> (0, 1=w370:i16[])
                  n220 = Wait (ms)(milliseconds to wait=u32 50) -> ()  [unwired: 1 out]
                  n221 = local read "already calibrated?"() -> (w362:bool)
                  n222 = property on="normalized spectra" class="XYGraph (strikt)"() -> ("CrsrList"=w360:T10)  [unwired: 2 in, 2 out]
                  n223 = Array Max & Min(array=w370) -> (max index (indices)=w371:i32)  [unwired: 3 out]
                  n224 = property on="Full Chip Plot" class="IntGraph (strikt)"() -> ("CrsrLis"=w359:T10)  [unwired: 2 in, 2 out]
                  n225 = Replace Array Subset(array=w368, new element=w361, index=w371) -> (w350:cluster{dbl[], dbl[]}[])
                  n226 = Build Array("First Edge [eV]", "Second Edge [eV]") -> (w347:dbl[])
                  n227 = call "Calibration.vi"("Full Chip Cursor List"=w359, "already calibrated?"=w362, "Calibrate IN"="Calibrate", "Input Plots"=w350, "Spectra Cursor List"=w360, "Edges"=w347, "Energy scale IN"=w346) -> ("label x-axis"=w363:string, "Output Plots"=w364:cluster{dbl[], dbl[]}[], "Energy scale in eV"=w345:dbl[], "already calibrated? OUT"=w354:bool)  [unwired: 1 in]
                  "Energy Scale in eV" <- w345
                  n228 = case shown="False" w369 {
                    tunnel: w364 -> [w397 _]
                    tunnel: w343 -> [w398 _]
                    tunnel: w337 -> [w396 _]
                    tunnel: w351 -> [w395 _]
                    tunnel: w338 -> [w394 _]
                    tunnel: w359 -> [w393 _]
                    tunnel: w363 -> [w392 _]
                    tunnel: w354 -> [w391 _]
                    tunnel: w345 -> [w390 _]
                    frame False {
                      n229 = stacked-sequence {
                        tunnel: w398 -> [_ _ _ w439]
                        tunnel: w395 -> [_ _ _ w438]
                        tunnel: w397 -> [_ _ _ w433]
                        tunnel: w396 -> [_ _ _ w435]
                        tunnel: w394 -> [_ _ _ w434]
                        tunnel: w393 -> [_ w414 _ _]
                        tunnel: w392 -> [_ _ w427 _]
                        tunnel: w391 -> [_ _ _ w431]
                        tunnel: w390 -> [_ _ _ w430]
                        frame #0 {
                          n230 = Number To Boolean Array(number="calibration spectra") -> (Boolean array=w403:bool[])
                          n231 = Index Array(array=w403, index #1=0 ("index"), index #2=1 ("index"), index #3=2 ("index")) -> (element #1=w404:bool, element #2=w405:bool, element #3=w406:bool)
                          n232 = property on="current spectrum" class="XYGraph (strikt)"("Visible"=w404) -> ()  [unwired: 2 in, 2 out]
                          n233 = property on="averaged spectrum" class="XYGraph (strikt)"("Visible"=w405) -> ()  [unwired: 2 in, 2 out]
                          n234 = property on="background spectrum" class="XYGraph (strikt)"("Visible"=w406) -> ()  [unwired: 2 in, 2 out]
                        }
                        frame #1 {
                          w415 = u32 1 items=["1"=1, "2"=2, "4"=4, "10"=10] ("Binning 1")
                          n235 = local read "Use Cursors"() -> (w412:bool)
                          n236 = local read "Binning 1"() -> (w409:u32)
                          n237 = call "Round_Min_Max.vi"("Binning 1"=w415, "CrsList"=w414, "Use Cursors"=w412) -> ("min(X)"=w410:u32, "max(X)"=w411:u32)  [unwired: 5 in, 2 out]
                          n238 = case shown="True" w412 {
                            tunnel: w411 -> [w418 w421]
                            tunnel: w410 -> [w417 w422]
                            tunnel: w409 -> [_ w423]
                            tunnel: [w417 w420] -> w407
                            tunnel: [w418 w419] -> w408
                            frame False {
                            }
                            frame True {
                              n239 = Multiply(x=w423, y=w421) -> (x*y=w419:u32)
                              n240 = Multiply(x=w422, y=w423) -> (x*y=w420:u32)
                            }
                          }
                          n241 = property on="normalized spectra" class="XYGraph (strikt)"("XScale.NameLbl.Text"="Pixel" ("X-Achse.Namensbeschriftung.Text"), "XScale.Maximum"=w408, "XScale.Minimum"=w407, "XScale.ScaleFit"=u8 0 ("X Scale.Scale Fit")) -> ()  [unwired: 2 in, 2 out]
                        }
                        frame #2 {
                          w426 = u8 2 ("X Scale.Scale Fit")
                          n242 = case shown="True" "Autoscale" {
                            tunnel: [u8 0 ("X Scale.Scale Fit") u8 2 ("X Scale.Scale Fit")] -> w425
                            frame False {
                            }
                            frame True {
                            }
                          }
                          n243 = property on="current spectrum" class="XYGraph (strikt)"("XScale.NameLbl.Text"=w427, "XScale.ScaleFit"=w426, "YScale.ScaleFit"=w425) -> ()  [unwired: 2 in, 2 out]
                          n244 = property on="averaged spectrum" class="XYGraph (strikt)"("XScale.NameLbl.Text"=w427, "XScale.ScaleFit"=w426, "YScale.ScaleFit"=w425) -> ()  [unwired: 2 in, 2 out]
                          n245 = property on="background spectrum" class="XYGraph (strikt)"("XScale.NameLbl.Text"=w427, "XScale.ScaleFit"=w426, "YScale.ScaleFit"=w425) -> ()  [unwired: 2 in, 2 out]
                        }
                        frame #3 {
                          n246 = Select(t=w430, s=w431, f=w438) -> (s? t:f=w440:dbl[])
                          n247 = Bundle("pixel scale"=w440, "output spectrum"=w434) -> (w441:T14)  [unwired: 1 in]
                          n248 = Bundle("pixel scale"=w440, "background\nspectrum"=w439) -> (w442:T15)  [unwired: 1 in]
                          n249 = Bundle("pixel scale"=w440, "output spectrum"=w435) -> (w443:T14)  [unwired: 1 in]
                          n250 = Build Array(w441) -> (→"current spectrum":T5)
                          n251 = Build Array(w442) -> (→"background spectrum":T16)
                          n252 = Build Array(w443) -> (→"averaged spectrum":T5)
                          "normalized spectra" <- w433
                        }
                      }
                    }
                    frame True {
                    }
                  }
                  n253 = stacked-sequence {
                    tunnel: w354 -> [w385 _ _]
                    frame #0 {
                      "already calibrated?" <- w385
                    }
                    frame #1 {
                      n254 = case shown="True" "New Calibration" {
                        frame False {
                        }
                        frame True {
                          n255 = local write "already calibrated?"(FALSE) -> ()
                        }
                      }
                    }
                    frame #2 {
                      n256 = case shown="True" "Use latest\nEnergy Scale" {
                        frame False {
                        }
                        frame True {
                          n257 = local write "already calibrated?"(TRUE) -> ()
                        }
                      }
                    }
                  }
                }
              }
            }
          }
          event "Start Measurement": Value Change {
            n258 = event-data() -> ()  [unwired: 1 in, 6 out]
            n259 = stacked-sequence {
              frame #0 {
                w446 = u32 1 items=["1"=1, "2"=2, "4"=4, "10"=10] ("Binning 1")
                n260 = local read "Integration Time [s]"() -> (w456:dbl)
                n261 = Bundle By Name(cluster=T8 {"X start"=1, "X end"=1340, "X Binning/Grouping"=1, "Y start"=1, "Y end"=400, "Y Binning/Grouping"=400} ("ROI Parameters"), "X Binning/Grouping"=w446) -> (w449:T8)
                n262 = Divide(x=u32 1340, y=w446) -> (x/y=w447:dbl)
                n263 = local read "Image Handle"() -> (w452:u32)
                n264 = local read "Parameters"() -> (w455:T6)
                n265 = local write "Substract\nBackground 3"(FALSE ("Substract\nBackground 3")) -> ()
                n266 = for {
                  N: w447 -> [_]
                  tunnel: [w457] -> w445 mode=indexing
                  i -> [w457]
                }
                n267 = call "Init_Camera.vi"("Binning IN"=w446, "Use Cursors IN"=FALSE ("Full Chip IN"), "Image Handle IN"=w452, "ROI Parameters"=w449, "integration time [s]"=w456, "Parameters IN"=w455) -> ("Image Handle OUT"=w453:u32, "Parameters OUT"=w454:T6)  [unwired: 4 in]
                n268 = local write "Parameters"(w454) -> ()
                n269 = local write "Image Handle"(w453) -> ()
                n270 = local write "pixel scale"(w445) -> ()
              }
              frame #1 {
                n271 = local read "background\nspectrum"() -> (w463:dbl[])
                n272 = Initialize Array(0.0 ("element"), 10 ("Dimension"), 1340 ("dimension size")) -> (w459:dbl[][])
                n273 = while {
                  shift-right: [w470] -> _
                  shift-left: w459 -> [w472]
                  shift-right: [w471] -> _
                  shift-left: 1 -> [w475]
                  tunnel: w463 -> [w484]
                  stop <- w489 stop-if-true
                  w482 = u32 1 items=["1"=1, "2"=2, "4"=4, "10"=10] ("Binning 1")
                  w488 = u16 1 items=["array", "spectrum"] ("average")
                  n274 = local read "Leave Program"() -> (w495:bool)
                  n275 = local read "Parameters"() -> (w497:T6)
                  n276 = local read "Image Handle"() -> (w496:u32)
                  n277 = call "Read_Camera.vi"("data type"=w488, "Image Handle IN"=w496, "input parameters"=w497) -> ("spectrum"=w485:dbl[], "output parameters"=w498:T6, "exit program"=w493:bool)  [unwired: 4 in, 2 out]
                  n278 = Compound Arithmetic op=OR(w493, "stop 4", w495) -> (w489:bool)
                  n279 = local read "Use Cursors"() -> (w479:bool)
                  n280 = property on="Full Chip Plot" class="IntGraph (strikt)"() -> ("CrsrLis"=w491:T10)  [unwired: 2 in, 2 out]
                  n281 = local read "Binning 1"() -> (w481:u32)
                  n282 = local write "Parameters"(w498) -> ()
                  n283 = Not(x=w489) -> (.not. x?=w490:bool)
                  n284 = local write "Start Measurement"(w490) -> ()
                  n285 = call "Round_Min_Max.vi"("Binning 1"=w482, "CrsList"=w491, "Use Cursors"=w479) -> ("min(X)"=w476:u32, "max(X)"=w480:u32)  [unwired: 5 in, 2 out]
                  n286 = case shown="True" w479 {
                    tunnel: w480 -> [w519 w523]
                    tunnel: w481 -> [_ w524]
                    tunnel: [w518 w522] -> w478
                    tunnel: [w519 w521] -> w477
                    tunnel: w476 -> [w518 w520]
                    frame False {
                    }
                    frame True {
                      n287 = Multiply(x=w524, y=w523) -> (x*y=w521:u32)
                      n288 = Multiply(x=w520, y=w524) -> (x*y=w522:u32)
                    }
                  }
                  n289 = call "Substract_Spectrum.vi"("Substract Background"="Substract\nBackground 3", "spectrum"=w485, "background spectrum"=w484) -> ("output spectrum"=w473:dbl[])  [unwired: 7 in]
                  n290 = Wait (ms)(milliseconds to wait=u32 50) -> ()  [unwired: 1 out]
                  n291 = call "Real_Average.vi"("new input spectrum"=w473, "old input array"=w472, "Number of averages"="Number \nof Averages", "current measurement number"=w475) -> ("output array"=w470:dbl[][], "next measurement number"=w471:i32, "output spectrum"=w466:dbl[])  [unwired: 5 in]
                  "Current\n Loop" <- w471
                  n292 = case shown="True" "Save to Logbook" {
                    frame False {
                    }
                    frame True {
                      w511 = u8 0 ("R")
                      n293 = control-ref of="XUV spectra measurement"() -> (w507:refnum<vi>)
                      n294 = call <vilib>:"RGB to Color.vi"("B"=w511, "G"=w511, "R"=w511) -> ("Color"=w512:u32)
                      n295 = invoke on="Methodenknoten" class="XYGraph (strikt)" method="Bild lesen"(reference=w507, "image depth"=8 ("Image Depth"), "bg color"=w512) -> ("image data"=w513:T13)  [unwired: 3 in, 5 out]
                      n296 = call <vilib>:"Write PNG File.vi"("image data"=w513, "path to PNG file"=path "temp.png") -> ("path"=w508:path)  [unwired: 8 in, 1 out]
                      n297 = local read "Integration Time [s]"() -> (w504:dbl)
                      n298 = Number To Fractional String(number=w504, precision (6)=2) -> (F-format string=w505:string)  [unwired: 2 in]
                      n299 = Concatenate Strings("Integration time: " ("String"), w505, "\r\n", "Comment") -> (w501:string)
                      n300 = call "sendtolabbook.vi"("File"=w508, "Text"=w501) -> ()  [unwired: 9 in, 1 out]
                    }
                  }
                  n301 = case shown="False" "Energy/Pixel" {
                    tunnel: [w515 w517] -> w469
                    tunnel: ["Energy [eV]" ("X Scale.Name Label.Text") "Pixel" ("X Scale.Name Label.Text")] -> w467
                    frame False {
                      n302 = local read "Energy Scale in eV"() -> (w515:dbl[])
                    }
                    frame True {
                      n303 = local read "pixel scale"() -> (w517:dbl[])
                    }
                  }
                  n304 = Subtract(x=w477, y=w478) -> (x-y=w492:u32)
                  n305 = Array Subset(array=w469, index=w478, length=w492) -> (w465:dbl[])
                  n306 = Build Array(w465, w466) -> (w487:dbl[][])
                  n307 = call "Save_2D_Array.vi"("Array"=w487, "Save"="Save Spectrum") -> ()  [unwired: 10 in]
                  n308 = stacked-sequence {
                    tunnel: w467 -> [w527 _]
                    tunnel: w466 -> [_ w536]
                    tunnel: w465 -> [_ w531]
                    frame #0 {
                      n309 = case shown="True" "Autoscale Spectrum" {
                        tunnel: [u8 0 ("X Scale.Scale Fit") u8 2 ("X Scale.Scale Fit")] -> w526
                        frame False {
                        }
                        frame True {
                        }
                      }
                      n310 = property on="XUV spectra measurement" class="XYGraph (strikt)"("XScale.NameLbl.Text"=w527, "XScale.ScaleFit"=u8 2 ("X-Achse.Achsenanpassung"), "YScale.ScaleFit"=w526) -> ()  [unwired: 2 in, 2 out]
                    }
                    frame #1 {
                      n311 = property on="XUV spectra measurement" class="XYGraph (strikt)"() -> ("Cursor.Cursor X"=w532:dbl)  [unwired: 2 in, 2 out]
                      n312 = call "Normalize_3.vi"("CursorX"=w532, "Energy Scale in eV"=w531, "raw data"=w536, "Normalize"="Normalize") -> ("Counts at X"=→"Counts at Cursor":dbl, "raw data"=w535:dbl[], "Max. Wert"=→"Max. Counts":dbl)  [unwired: 3 in]
                      n313 = Bundle(w531, "raw data"=w535) -> (w538:cluster{dbl[], "raw data":dbl[]})  [unwired: 1 in]
                      n314 = Build Array(w538) -> (→"XUV spectra measurement":cluster{dbl[], "raw data":dbl[]}[])
                    }
                  }
                }
              }
            }
          }
          event "Force Camera to Close": Value Change {
            n315 = event-data() -> ()  [unwired: 1 in, 6 out]
            n316 = local read "Parameters"() -> (w541:T6)
            n317 = Unbundle By Name(w541) -> ("camera parameters.Camera Handle"=w540:u32)
            n318 = call <userlib>:"CameraClose.vi"("error in"="error in", "Camera Handle"=w540) -> ("error out"=w544:errorcluster)
            n319 = call <userlib>:"UninitToolkit.vi"("error in"=w544) -> ("error out"=→"error out":errorcluster)
          }
          event "Destroy all Images": Value Change {
            n320 = event-data() -> ()  [unwired: 1 in, 6 out]
            n321 = for {
              N: 99 -> [_]
              i -> [w546]
              n322 = call <userlib>:"ImageDestroy.vi"("error in"="error in", "Data handle"=w546) -> ("error out"=→"error out":errorcluster)
            }
          }
          event "Leave Program": Value Change {
            n323 = event-data() -> ()  [unwired: 1 in, 6 out]
          }
        }
      }
    }
    frame #2 {
      # "Unitialise Camera and SIToolkit"
      n324 = local read "Parameters"() -> (w555:T6)
      n325 = local write "Leave Program"(FALSE ("Leave program")) -> ()
      n326 = Unbundle By Name(w555) -> ("camera parameters"=w556:T9, "error"=w553:errorcluster)
      n327 = Unbundle By Name(w556) -> ("Camera Handle"=w552:u32)
      n328 = call <userlib>:"CameraStop.vi"("error in"=w553, "Camera Handle"=w552) -> ("error out"=w551:errorcluster, "Camera Handle"=w550:u32)
      n329 = call <userlib>:"CameraClose.vi"("error in"=w551, "Camera Handle"=w550) -> ("error out"=w558:errorcluster)
      n330 = call <userlib>:"UninitToolkit.vi"("error in"=w558) -> ("error out"=w557:errorcluster)
      n331 = Bundle By Name(cluster=w555, "camera parameters"=w556, "error"=w557) -> (w554:T6)
      n332 = local write "Parameters"(w554) -> ()
    }
  }
  n333 = property on="Tab Control" class="RKElem (strikt)"("Auto Grow?"=FALSE) -> ()  [unwired: 2 in, 2 out]
